vi "AGG MISURE EL NM.vi"(6 "ACQ RESISTOMAT?":bool=TRUE, 7 "Cluster INFO":T26={"Scelta wattmetro"={"Wattmetro"=enum."No Selection"}, "SET RPM"=0.0, "SET TEMP"=0.0, "Array banchi"=[{"Nome"="Elettropompa", "Tors. scala1"=0, "Tors. scala2"=0, "rpm"=0, "TAMB"=0, "Indici Temperature"=[0, 1], "Indice freno"=1, "alimentatore trifase"=0, "alimentatore monofase"=0, "alimentatore dc arm"=0, "alimentatore dc ecc"=0, "alimentatore dc mp"=0}, {"Nome"="Sommersa", "Tors. scala1"=0, "Tors. scala2"=0, "rpm"=0, "TAMB"=1, "Indici Temperature"=[0, 1], "Indice freno"=0, "alimentatore trifase"=0, "alimentatore monofase"=0, "alimentatore dc arm"=0, "alimentatore dc ecc"=0, "alimentatore dc mp"=0}], "Array valvole linee avvio/fermata"=[], "banco selezionato"=0, "Nomi valvole prop sistema"=[], "canale-- sensore"=[], "Attriti B1"=[], "Attriti B2"=[], "Collegamento elettrico"={"ALIMENTAZIONE ELETTRICA"=enum."AC TRIFASE", "ID"=0, "#rami freddo\\eq term resmeter"=0, "#rami riscaldamento resmeter"=0, "#rami freddo\\eq term resistomat"=0, "#rami riscaldamento resistomat"=0, "CALCOLI"=enum."AC TRIFASE"}, "lingua"=0, "Costanti collaudo"={"P [bar]"=0.0, "T amb. [°C]"=0.0, "Umidità [%]"=0.0, "T acqua [°C] 2"=0.0}, "OPZIONI MISURE RES"={"MISURA A FREDDO"=enum."RESISTOMAT", "MISURA EQ. TERMICO"=enum."RESISTOMAT", "MISURA DT PROVA IN CORSO"=enum."RESISTOMAT - CON FERMATE", "MISURE PRIMA E DOPO"=enum."RESISTOMAT", "STRUMENTI PRESENTI"=enum."NESSUNO"}, "Dati targa motore"={"Vnom"=0.0, "Fnom"=0.0, "Inom"=0.0, "Cnom"=0.0, "Npoli"=0.0, "Scorta 1"=0.0, "Scorta 2"=0.0, "Scorta 3"=0.0}}, 8 "RPM":dbl, 9 "tamb":dbl format="%#_13g", 10 "MISURE ALL":T1={"Cluster READ NI"={"AI (0-10V)"={"AI 0"=0.0, "AI 1"=0.0, "AI 2"=0.0, "AI 3"=0.0, "AI 4"=0.0, "AI 5"=0.0, "AI 6"=0.0, "AI 7"=0.0, "AI 8"=0.0, "AI 9"=0.0, "AI 10"=0.0, "AI 11"=0.0, "AI 12"=0.0, "AI 13"=0.0, "AI 14"=0.0, "AI 15"=0.0, "AI 16"=0.0, "AI 17"=0.0, "AI 18"=0.0, "AI 19"=0.0, "AI 20"=0.0, "AI 21"=0.0, "AI 22"=0.0, "AI 23"=0.0, "AI 24"=0.0, "AI 25"=0.0, "AI 26"=0.0, "AI 27"=0.0, "AI 28"=0.0, "AI 29"=0.0, "AI 30"=0.0, "AI 31"=0.0}, "StatoAO_Cdaq[0-10V]"={"AO 1"=0.0, "AO 2"=0.0, "AO 3"=0.0, "AO 4"=0.0}, "Contatori [rpm]"={"RPM 1"=0.0, "RPM 2"=0.0}, "StatoAO_Cdaq [4-20mA]"={"Cdaq_AO [0-10V] 0 for Torque"=0.0, "Cdaq_AO [0-10V] 1"=0.0, "Cdaq_AO [0-10V] 2"=0.0, "Cdaq_AO [0-10V] 3"=0.0}, "StatoDO_Cdaq"={"Scorta 0"=FALSE, "Scorta 1"=FALSE, "Scorta 2"=FALSE, "Scorta 3"=FALSE, "Scorta 4"=FALSE, "Scorta 5"=FALSE, "Scorta 6"=FALSE, "Scorta 7"=FALSE, "Scorta 8"=FALSE, "Scorta 9"=FALSE, "Scorta 10"=FALSE, "Scorta 11"=FALSE, "Scorta 12"=FALSE, "Scorta 13"=FALSE, "Scorta 14"=FALSE, "Scorta 15"=FALSE, "Scorta 16"=FALSE, "Scorta 17"=FALSE, "Scorta 18"=FALSE, "Scorta 19"=FALSE, "Scorta 20"=FALSE, "Scorta 21"=FALSE, "Scorta 22"=FALSE, "Scorta 23"=FALSE, "Scorta 24"=FALSE, "Scorta 25"=FALSE, "Scorta 26"=FALSE, "Scorta 27"=FALSE, "Scorta 28"=FALSE, "Scorta 29"=FALSE, "Scorta 30"=FALSE, "Scorta 31"=FALSE}, "DI"={"Scorta 0"=FALSE, "Scorta 1"=FALSE, "Scorta 2"=FALSE, "Scorta 3"=FALSE, "Scorta 4"=FALSE, "Scorta 5"=FALSE, "Scorta 6"=FALSE, "Scorta 7"=FALSE, "Scorta 8"=FALSE, "Scorta 9"=FALSE, "Scorta 10"=FALSE, "Scorta 11"=FALSE, "Scorta 12"=FALSE, "Scorta 13"=FALSE, "Scorta 14"=FALSE, "Scorta 15"=FALSE, "Scorta 16"=FALSE, "Scorta 17"=FALSE, "Scorta 18"=FALSE, "Scorta 19"=FALSE, "Scorta 20"=FALSE, "Scorta 21"=FALSE, "Scorta 22"=FALSE, "Scorta 23"=FALSE, "Scorta 24"=FALSE, "Scorta 25"=FALSE, "Scorta 26"=FALSE, "Scorta 27"=FALSE, "Scorta 28"=FALSE, "Scorta 29"=FALSE, "Scorta 30"=FALSE, "Scorta 31"=FALSE}, "AI (4-20mA)"={"AI 0"=0.0, "AI 1"=0.0, "AI 2"=0.0, "AI 3"=0.0, "AI 4"=0.0, "AI 5"=0.0, "AI 6"=0.0, "AI 7"=0.0, "AI 8"=0.0, "AI 9"=0.0, "AI 10"=0.0, "AI 11"=0.0, "AI 12"=0.0, "AI 13"=0.0, "AI 14"=0.0, "AI 15"=0.0}, "TC [°C]"={"tc 1"=0.0, "tc 2"=0.0, "tc 3"=0.0, "tc 4"=0.0}, "NI Read Values"={"RPM"=0.0, "Frequency"=0.0, "Mod 1"={"Torsiometro 1"=0.0, "Torsiometro 2"=0.0, "Strin Gauge 1"=0.0, "Strin Gauge 2"=0.0}, "Mod 2"={"Termocoppia 1"=0.0, "Termocoppia 2"=0.0, "Termocoppia 3"=0.0, "Termocoppia 4"=0.0}, "Mod 3"={"PT 100 1"=0.0, "PT 100 2"=0.0, "PT 100 3"=0.0, "PT 100 4"=0.0}}}, "MISURE WT"={"URMS 1"=0.0, "IRMS 1"=0.0, "P 1"=0.0, "S 1"=0.0, "Q 1"=0.0, "LAMBDA 1"=0.0, "PHI 1"=0.0, "F U 1"=0.0, "F I 1"=0.0, "NONE 1"=0.0, "URMS 2"=0.0, "IRMS 2"=0.0, "P 2"=0.0, "S 2"=0.0, "Q 2"=0.0, "LAMBDA 2"=0.0, "PHI 2"=0.0, "F U 2"=0.0, "F I 2"=0.0, "NONE 2"=0.0, "URMS 3"=0.0, "IRMS 3"=0.0, "P 3"=0.0, "S 3"=0.0, "Q 3"=0.0, "LAMBDA 3"=0.0, "PHI 3"=0.0, "F U 3"=0.0, "F I 3"=0.0, "NONE 3"=0.0, "URMS SIGMA"=0.0, "IRMS SIGMA"=0.0, "P SIGMA"=0.0, "S SIGMA"=0.0, "Q SIGMA"=0.0, "LAMBDA SIGMA"=0.0, "PHI SIGMA"=0.0, "F U SIGMA"=0.0, "F I SIGMA"=0.0, "NONE 4"=0.0}, "Resistenze Resistomat"={"Res Ch1"=0.0, "Res Ch2"=0.0, "Res Ch3"=0.0, "Tamb"=0.0}, "INTERFACCIA"={"AI"={"Portate"=[], "Pressioni"=[], "Coppie[Nm]"=[], "Valvole prop %"=[], "RPM"=[], "Livelli"=[], "Temperature"=[], "Riferimenti %"=[], "TENSIONI"=[], "CORRENTI"=[]}, "DI (logici)"={"Start da pulsantiera"=FALSE, "Stop da pulsantiera"=FALSE, "Reset da pulsantiera"=FALSE, "Sistema OK"=FALSE, "Collaudo abilitato"=FALSE, "Potenza trifase abilitata"=FALSE, "Potenza monofase abilitata"=FALSE, "Potenza DC abilitata"=FALSE, "Potenza DC ECC abilitata"=FALSE, "Start alimentazione AC"=FALSE, "Start alimentazione DC"=FALSE, "Start DC eccitazione"=FALSE, "Teleruttore WT abilitato"=FALSE, "Teleruttore Resistomat abilitato"=FALSE, "Teleruttore corto fasi"=FALSE, "Ramo 1 resistomat"=FALSE, "Ramo 2 resistomat"=FALSE, "Ramo 3 resistomat"=FALSE, "B1 Scelta linea elettrica 1"=FALSE, "B1 Scelta linea elettrica 2"=FALSE, "B1 Scelta linea elettrica 3"=FALSE, "B1 Scelta linea elettrica 4"=FALSE, "B1 Scelta linea elettrica 5"=FALSE, "B2 Scelta linea elettrica 1"=FALSE, "B2 Scelta linea elettrica 2"=FALSE, "B2 Scelta linea elettrica 3"=FALSE, "B2 Scelta linea elettrica 4"=FALSE, "B2 Scelta linea elettrica 5"=FALSE, "Rotore bloccato 1"=FALSE, "Rotore bloccato 2"=FALSE, "FRENO 1 abilitato"=FALSE, "FRENO 1 run"=FALSE, "FRENO 1 senso rotaz"=FALSE, "FRENO 1 ctrl velocità"=FALSE, "FRENO 2 abilitato"=FALSE, "FRENO 2 run"=FALSE, "FRENO 2 senso rotaz"=FALSE, "FRENO 2 ctrl velocità"=FALSE, "ALIM 1 abilitato"=FALSE, "ALIM 1 run"=FALSE, "ALIM 2 abilitato"=FALSE, "ALIM 2 run"=FALSE, "ALIM 3 abilitato"=FALSE, "ALIM 3 run"=FALSE, "FRENO 1 ctrl coppia"=FALSE, "FRENO 2 ctrl coppia"=FALSE, "FRENO 3 ctrl coppia"=FALSE, "DI (logici) aggiuntivi impianto"={"Solo freno abilitato"=FALSE, "Carico resistivo abilitato"=FALSE, "AFE+freno abilitato"=FALSE, "Protezioni chiuse"=FALSE, "Start potenza AFE"=FALSE, "AFE in marcia"=FALSE}, "Misura corrente diretta WT"=FALSE, "Misura corrente sens ext"=FALSE, "Sens ext abilitati"=FALSE}, "AO non scalati"={"FRENO1 rif vel"=0.0, "FRENO1 rif Coppia"=0.0, "FRENO2 rif vel"=0.0, "FRENO2 rif Coppia"=0.0, "ALIM1 rif V"=0.0, "ALIM1 rif F"=0.0, "ALIM2 rif V"=0.0, "ALIM2 rif F"=0.0, "ALIM3 rif V"=0.0, "ALIM3 rif F"=0.0, "Fnom keb"=0.0, "Rpm nom keb"=0.0, "Pnom keb"=0.0, "Inom keb"=0.0, "Vnom keb"=0.0, "Rpm max keb"=0.0, "Tempo rampa keb"=0.0, "Tipo Mot keb"=0.0, "FRENO  rif Coppia "=0.0, "FRENO  rif  Corrente"=0.0}, "AO scalati"={"FRENO1 rif vel"=0.0, "FRENO1 rif Coppia"=0.0, "FRENO2 rif vel"=0.0, "FRENO2 rif Coppia"=0.0, "ALIM1 rif V"=0.0, "ALIM1 rif F"=0.0, "ALIM2 rif V"=0.0, "ALIM2 rif F"=0.0, "ALIM3 rif V"=0.0, "ALIM3 rif F"=0.0, "Fnom keb"=0.0, "Rpm nom keb"=0.0, "Pnom keb"=0.0, "Inom keb"=0.0, "Vnom keb"=0.0, "Rpm max keb"=0.0, "Tempo rampa keb"=0.0, "Tipo Mot keb"=0.0, "FRENO  rif Coppia "=0.0, "FRENO  rif  Corrente"=0.0}, "DO (logici)"={"Scelta banco 1"=FALSE, "Scelta banco 2"=FALSE, "Scelta banco 3"=FALSE, "FRENO 1 abilita"=FALSE, "FRENO 1 start"=FALSE, "FRENO 1 senso rotaz"=FALSE, "FRENO 1 ctrl velocità"=FALSE, "FRENO 2 abilita"=FALSE, "FRENO 2 start"=FALSE, "FRENO 2 senso rotaz"=FALSE, "FRENO 2 ctrl velocità"=FALSE, "ALIM 1 abilita"=FALSE, "ALIM 1 start"=FALSE, "ALIM 2 abilita"=FALSE, "ALIM 2 start"=FALSE, "ALIM 3 abilita"=FALSE, "ALIM 3 start"=FALSE, "Abilita linea trifase"=FALSE, "Abilita linea monofase"=FALSE, "Abilita linea dc"=FALSE, "Abilita linea dc eccit"=FALSE, "B1 Linea elettrica 1"=FALSE, "B1 Linea elettrica 2"=FALSE, "B1 Linea elettrica 3"=FALSE, "B1 Linea elettrica 4"=FALSE, "B1 Linea elettrica 5"=FALSE, "B2 Linea elettrica 1"=FALSE, "B2 Linea elettrica 2"=FALSE, "B2 Linea elettrica 3"=FALSE, "B2 Linea elettrica 4"=FALSE, "B2 Linea elettrica 5"=FALSE, "Start potenza AC"=FALSE, "Stop pontenza AC"=FALSE, "Start potenza DC"=FALSE, "Stop potenza DC"=FALSE, "Start potenza eccitaz"=FALSE, "Stop potenza eccitaz"=FALSE, "Reset allarmi"=FALSE, "watchdog"=FALSE, "Scala torsiometro B1"=FALSE, "Controllo torsiom B1"=FALSE, "Scala torsiometro B2"=FALSE, "Controllo torsiom B2"=FALSE, "Teleruttore WT abilita"=FALSE, "Teleruttore Resistomat abilita"=FALSE, "Teleruttore corto fasi"=FALSE, "Ramo 1 resistomat"=FALSE, "Ramo 2 resistomat"=FALSE, "Ramo 3 resistomat"=FALSE, "Collaudo in corso"=FALSE, "Allarme presente"=FALSE, "Enable Res Meter"=FALSE, "Bypass Res Meter"=FALSE, "2nd canale Res Meter"=FALSE, "Scala 200/2000 res meter"=FALSE, "Taratura res meter"=FALSE, "FRENO 1 ctrl coppia"=FALSE, "FRENO 2 ctrl coppia"=FALSE, "FRENO 3 ctrl coppia"=FALSE, "Aggiuntivi impianto"={"Senso rotazione alim 1"=FALSE, "Senso rotazione alim 2"=FALSE}, "ALIM 1 stop"=FALSE, "ALIM 2 stop"=FALSE, "ALIM 3 stop"=FALSE, "FRENO 1 stop"=FALSE, "FRENO 2 stop"=FALSE, "FRENO 3 stop"=FALSE, "B1 configurazione freno B"=FALSE, "B2 configurazione freno B"=FALSE, "Abilita scrittura KEB"=FALSE, "Bench Selection (0-B1,1-B2)"=FALSE, "Select current mode"=FALSE, "Select torque mode"=FALSE, "Select speed mode"=FALSE, "Start"=FALSE, "Stop"=FALSE, "Block"=FALSE, "Enable Force mode"=FALSE, "Abilita linea 125 A"=FALSE, "Abilita linea 63 A"=FALSE, "Abilita linea 16 A"=FALSE, "Aum Tensione Variac"=FALSE, "Dim Tesnione Variac"=FALSE, "Abilita ellectro stractura"=FALSE, "Risprinito Emergence"=FALSE, "Abilita collaudo"=FALSE, "Disabilita collaudo"=FALSE, "External Alaram"=FALSE, "Enable external program"=FALSE, "Reset"=FALSE, "Abilita Ingresso Variac"=FALSE, "Abilita Ventilatore Variac"=FALSE, "Abilita Uscita Variac "=FALSE}}, "FREDDO resistomat"={"Res Ch1"=0.0, "Res Ch2"=0.0, "tAMB"=0.0, "Res Ch3"=0.0}, "STATO PLC 1"={"USCITE PLC"={"AO (real) 2"={"SCORTA 1"=0.0, "SCORTA 2"=0.0, "SCORTA 3"=0.0, "SCORTA 4"=0.0, "SCORTA 5"=0.0, "SCORTA 6"=0.0, "SCORTA 7"=0.0, "SCORTA 8"=0.0}, "statoAO_PLC out"={"Rif Lim coppia freno [%]"=nan, "Rif rpm freno [%]"=nan, "Rif coppia freno [%]"=0.0, "Rif V alimentatore [%]"=0.0, "Rif F alimentatore [%]"=0.0}, "DO (bit)"={"Scelta banco 1"=FALSE, "Set dati motore freno 2"=FALSE, "Diretto inverter"=FALSE, "Filtro LC"=FALSE, "Marcia ALIM (1s)"=FALSE, "Marcia FRENO (1s)"=FALSE, "Stop AFE (1s)"=FALSE, "Stop freno (1s)"=FALSE, "Reset allarmi"=FALSE, "Watchdog"=FALSE, "Senso rotazione"=FALSE, "Abilita collaudo (1s)"=FALSE, "Disabilita collaudo (1s)"=FALSE, "Abilitazione ALIM"=FALSE, "Abilitazione FRENO"=FALSE, "Teleruttore WT"=FALSE, "Senso rot motore prova"=FALSE, "Scorta 7"=FALSE, "Scorta 8"=FALSE, "Scorta 9"=FALSE, "Scorta 10"=FALSE, "Scorta 11"=FALSE, "Scorta 12"=FALSE, "Scorta 13"=FALSE}}, "Stato DI_PLC"={"Sistema OK"=FALSE, "Rotore bloccato"=FALSE, "Scorta 1"=FALSE, "Prova diretto inverter"=FALSE, "Prova con filtro LC"=FALSE, "Teleruttore WT abilitato"=FALSE, "Alim sinus penta abilitato"=FALSE, "Alim sinus penta in marcia"=FALSE, "Freno abilitato"=FALSE, "Freno in marcia"=FALSE, "Senso rotazione freno"=FALSE, "Potenza abilitata"=FALSE, "Scorta 3"=FALSE, "Scorta 4"=FALSE, "scorta 5"=FALSE, "scorta 6"=FALSE}, "AI plc"={"Allarmi 1"=0.0, "Allarmi 2"=0.0, "Scorta 1"=0.0, "Scorta 2"=0.0, "RPM mot prova"=0.0, "I mot prova"=0.0, "RPM freno"=0.0, "I freno"=0.0, "Scorta 3"=0.0, "Scorta 4"=0.0}}, "Res Ch2"=0.0, "Res Ch2 2"=0.0, "FREDDO res meter"={"Res Ch1"=0.0, "Res Ch2"=0.0, "tAMB"=0.0, "Res Ch3"=0.0}, "Resistenze Res Meter"={"Res Ch1"=0.0, "Res Ch2"=0.0, "Res Ch3"=0.0, "Tamb"=0.0}, "READ SINUS PENTA"={"Menù Misure motore (M000-M030)"={"Rif vel a regime (int)"=0, "Rif vel a regime (dec)"=0, "Rif vel dopo rampe (int)"=0, "Rif vel dopo rampe (dec)"=0, "RPM motore (int)"=0, "RPM motore (dec)"=0, "FREQout inverter"=0, "Rif coppia a regime(Nm)"=0, "Richiesta di coppia (Nm)"=0, "Coppia generata dal motore(Nm)"=0, "Rif coppia a regime(%)"=0, "Richiesta di coppia (%)"=0, "Coppia generata dal motore(%)"=0, "Coppia max richiesta prima delle rampe(Nm)"=0, "Coppia max richiesta dopo le rampe(Nm)"=0, "Limite di velocità prima delle rampe"=0, "Limite di velocità dopo le rampe"=0, "Coppia max richiesta prima delle rampe(%)"=0, "Coppia max richiesta dopo le rampe(%)"=0, "Rif di flusso"=0, "Corrente di uscita"=0, "Capacità termica del motore"=0, "Tensione di uscita"=0, "Potenza di uscita"=0, "Energia consumata (LSword)"=0, "Energia consumata (MSword)"=0, "Tensione bus DC"=0, "Tensione di rete"=0}, "Menù regolatore PID (M018-M024)"={"Rif PID a regime(%)"=0, "Rif pid dopo rampe(%)"=0, "Retroazione del pid(%)"=0, "Errore del pid(%)"=0, "uscita del pid(%)"=0, "Rif del pid dopo le rampe"=0, "Retroazione del pid"=0}, "Menù ingressi digitali (M031-M036)"={"Ingressi digitali ritardati"=0, "Ingressi digitali istantanei"=0, "Moresettiera comando loc"=0, "Morsett comando da seriale"=0, "Morsett comando bus di campo"=0, "Ing dig ausiliari da morsettiera"=0, "Ing dig ausiliari da seriale"=0}, "Menù riferimenti (M037-M051)"={"Rif analog est REF"=0, "Rif analog est AIN1"=0, "Rif analog est AIN2"=0, "Rif analog est XAIN4"=0, "Rif analog est XAIN5"=0, "Rif velocità da seriale(int)"=0, "Rif velocità bus di campo(int)"=0, "Rif coppia da seriale"=0, "Rif coppia bus di campo"=0, "Rif del PID da seriale"=0, "Rif del PID da bus di campo"=0, "Retroazione del PID da seriale"=0, "Retroazione del PIDda bus di campo"=0, "Rif da encoder"=0, "Rif in frequenza"=0, "Rif velocità da seriale(dec)"=0, "Rif velocità bus di campo(dec)"=0}, "Menù rampe (P009-P033)"={"Tempo di dec rampa di vel 1"=0, "Tempo di acc rampa di vel 2"=0, "Tempo di dec rampa di vel 2"=0, "Tempo di acc rampa di vel 1"=0, "Unità di mis tempi rampe vel 1/2"=0, "Tempo di acc rampa di vel 3"=0, "Tempo di dec rampa di vel 3"=0, "Tempo di acc rampa di vel 4"=0, "Tempo di dec rampa di vel 4"=0, "Unità di mis tempi rampe vel 3/4"=0, "Selettore arrottondam rampe"=0, "Tempo di arrotond iniz rampa acc"=0, "Tempo di arrotond finale rampa acc"=0, "Tempo di arrotond iniz rampa dec"=0, "Tempo di rampa di salita rif coppia"=0, "Tempo di rampa di discesa rif coppia"=0, "Unità di misura rampa coppia"=0, "Tempo rampa acc marcia jog"=0, "Tempo rampa dec marcia jog"=0, "Reset acc ai cambi pendenza"=0, "rampa di acc in fire mode"=0, "rampa di dec in fire mode"=0, "Tempo di arrotond finale rampa dec"=0}, "Menù controllo motore(C008-C128)"={"Numero motori configurati"=0, "Tipo algoritmo di controllo Mot1"=0, "Tipo rif Mot1"=0, "Tensione nominale rete"=0, "Retroaz di vel da encoder Mot1"=0, "Tipo curva V/f Mot1"=0, "Rotazione delle fasi Mot1"=0, "Freq nominale del motore Mot1"=0, "RPM nominali del motore Mot1"=0, "Potenza nominale del motore Mot1"=0, "Corrente nominale del motore Mot1"=0, "Tensione nominale del motore mot1"=0, "Potenza a vuoto del motore Mot1"=0, "Corrente a vuoto del motore Mot1"=0, "Resistenza statorica del motore Mot1"=0, "Induttanza di dispersione Mot1"=0, "Induttanza mutua motore"=0, "Costante di tempo rotorica"=0, "Costante di tempo filtro pb"=0, "Velocità minima motore"=0, "Velocità massima motore"=0}, "Menù configurazione PID"={"Selezione riferimento n.1"=0, "Selezione retroazione n.1"=0, "Modalità di fuzionamento PID"=0, "Termine derivativo calcolato su err o mis"=0, "Proporz moltiplica deriv e integrale"=0, "Azione del PID"=0}, "ID"=0.0, "Menù uscite digitali"={"MDO4 Inverter pronto"=0}, "Fcarrier"={"Fcarrier Min (Hz)"=0, "Fcarrier Max (Hz)"=0}, "stato inverter M089"=0.0, "Riferimenti"={"Rif tensione"=0, "Rif velocità"=0}, "Comunicazione"=FALSE, "Modalità stop"=0.0}, "STATO PLC 2"={"USCITE PLC"={"AO (real) 2"={"SCORTA 1"=0.0, "SCORTA 2"=0.0, "SCORTA 3"=0.0, "SCORTA 4"=0.0, "SCORTA 5"=0.0, "SCORTA 6"=0.0, "SCORTA 7"=0.0, "SCORTA 8"=0.0}, "statoAO_PLC out"={"Condensatori"=0.0, "Scorta 1"=0.0, "Scorta 2"=0.0}, "DO (bit)"={"Relè misura resistomat"=FALSE, "Misura res ramo 1"=FALSE, "Misura res ramo 2"=FALSE, "Misura res ramo 3"=FALSE, "Scelta banco 2"=FALSE, "Scala Torsiometro"=FALSE, "Ctrl torsiometro"=FALSE, "Select current mode"=FALSE, "Select Torque mode"=FALSE, "Select speed mode"=FALSE, "Watchdog"=FALSE, "Scorta"=FALSE, "Scorta 2"=FALSE, "Scorta 3"=FALSE, "Scorta 4"=FALSE, "Scorta 5"=FALSE, "Bench selection"=FALSE, "External alarm"=FALSE, "Enable external program"=FALSE, "Reset allarmi"=FALSE, "Start"=FALSE, "Stop"=FALSE, "Block"=FALSE, "Scorta 6"=FALSE}}, "Stato DI_PLC"={"Sistema ok"=FALSE, "Relè Resistomat abilitato"=FALSE, "Freno abilitato"=FALSE, "Freno in marcia"=FALSE, "scorta b"=FALSE, "scorta a"=FALSE, "scorta 1"=FALSE, "scorta 2"=FALSE, "scorta 3"=FALSE, "scorta 4"=FALSE, "Scorta 5"=FALSE, "Scorta 6"=FALSE, "Scorta 7"=FALSE, "Scorta 8"=FALSE, "Scorta 9"=FALSE, "Scorta 10"=FALSE}, "AI plc"={"Allarmi 1"=0.0, "Allarmi 2"=0.0, "TC 1"=0.0, "TC 2"=0.0, "TC 3"=0.0, "TC 4"=0.0, "TC 5"=0.0, "TC 6"=0.0, "TC 7"=0.0, "TC 8"=0.0, "PT1000 1"=0.0, "PT1000 2"=0.0, "PT1000 3"=0.0, "PT1000 4"=0.0}}, "STATO PLC 3"={"USCITE PLC"={"AO (real) 2"={"SCORTA 1"=0.0, "SCORTA 2"=0.0, "SCORTA 3"=0.0, "SCORTA 4"=0.0, "SCORTA 5"=0.0, "SCORTA 6"=0.0, "SCORTA 7"=0.0, "SCORTA 8"=0.0}, "statoAO_PLC out"={"Rif velocità alimentatore"=0.0, "Scorta"=0.0, "Tipo Motore  keb"=0.0, "I nom keb"=0.0, "RPM nom keb"=0.0, "V nom keb"=0.0, "F nom keb"=0.0, "t rampa keb"=0.0}, "DO (bit)"={"Select linea Inverter"=FALSE, "Abilita sense wattmetro"=FALSE, "Bypass filtro LC"=FALSE, "Filtro LC"=FALSE, "Bypass trasformatore"=FALSE, "Trasformatore"=FALSE, "Abilita uscite variac"=FALSE, "Abilita linea 125 A"=FALSE, "Abilita linea 63 A"=FALSE, "Abilita linea 16 A"=FALSE, "Abilita Scrittura Dati Keb"=FALSE, "Abilita alimentatore"=FALSE, "Marcia alimentatore (1s)"=FALSE, "Stop alimentatore (1s)"=FALSE, "Senso rot mot prova"=FALSE, "Watchdog"=FALSE, "Aumenta tensione variac"=FALSE, "Diminuisci tensione variac "=FALSE, "Blocco elettroserrature"=FALSE, "Ripristino emergence"=FALSE, "Abilita ingresso variac"=FALSE, "Abilita ventilatore variac"=FALSE, "Reset Allarm"=FALSE, "Scorta 1"=FALSE, "Scorta 2"=FALSE, "Scorta 3"=FALSE, "Scorta 4"=FALSE, "Scorta 5"=FALSE, "Scorta 6"=FALSE, "Scorta 7"=FALSE, "Scorta 8"=FALSE, "Scorta 9"=FALSE, "Abilita collaudo"=FALSE, "Disabilita collaudo "=FALSE, "Scorta 10"=FALSE, "Scorta 11"=FALSE, "Scorta 12"=FALSE, "Scorta 13"=FALSE, "Scorta 14"=FALSE, "Scorta 15"=FALSE}}, "Stato DI_PLC"={"Sistema OK"=FALSE, "Rotore bloccato"=FALSE, "Filtro LC"=FALSE, "Bypass Filtro LC"=FALSE, "Scelta Trasformatore"=FALSE, "Scelta Bypass trasformatore"=FALSE, "Teleruttore wt abilitato"=FALSE, "Alimentatore abilitato"=FALSE, "Alimentatore in marcia"=FALSE, "Scorta 1"=FALSE, "Scorta 2"=FALSE, "Scorta 3"=FALSE, "Potenza abilitata"=FALSE, "Alimentatore in allarme"=FALSE, "Scorta 4"=FALSE, "Conferma dati KEB"=FALSE, "Scorta 5"=FALSE, "Warning Inverter Alimentatore"=FALSE, "Variac Abilitato"=FALSE, "Linea 125 A abilitata"=FALSE, "Linea 63 A abilitata"=FALSE, "Linea 16 A abilitata"=FALSE, "Scorta 6"=FALSE, "Enable force mode"=FALSE}, "AI plc"={"Allarmi 1"=0.0, "Allarmi 2"=0.0, "RPM motore prova"=0.0, "Corrente motore prova"=0.0, "RPM freno"=0.0, "Corrente freno"=0.0, "Tipo motore keb"=0.0, "I nom keb"=0.0, "RPM nom keb"=0.0, "V nom keb"=0.0, "F nom keb"=0.0, "T rampa keb"=0.0, "scorta"=0.0, "Scorta 2"=0.0}}, "DCREG"={"Parametri di misura"={"M000"=0.0, "M001"=0.0, "M002"=0.0, "M003"=0.0, "M004"=0.0, "M005"=0.0, "M006"=0.0, "M007"=0.0, "M008"=0.0, "M009"=0.0, "M010"=0.0, "M011"=0.0, "M012"=0.0, "M013"=0.0, "M014"=0.0, "M015"=0.0, "M016"=0.0, "M017"=0.0, "M018"=0.0, "M019"=0.0, "M020"=0.0, "M021"=0.0, "M022"=0.0, "M023"=0.0, "M024"=0.0, "M025"=0.0, "M026"=0.0, "M027"=0.0, "M028"=0.0, "M029"=0.0, "M030"=0.0, "M031"=0.0}, "Parametri di programmazione"={"P000"=0.0, "P001"=0.0, "P002"=0.0, "P003"=0.0, "P004"=0.0, "P005"=0.0, "P006"=0.0, "P010"=0.0, "P011"=0.0, "P012"=0.0, "P013"=0.0, "P014"=0.0, "P015"=0.0, "P016"=0.0, "P030"=0.0, "P031"=0.0, "P032"=0.0, "P033"=0.0, "P034"=0.0, "P035"=0.0, "P036"=0.0, "P037"=0.0, "P038"=0.0, "P039"=0.0, "P040"=0.0, "P050"=0.0, "P051"=0.0, "P052"=0.0, "P053"=0.0, "P054"=0.0, "P055"=0.0, "P056"=0.0, "P057"=0.0, "P058"=0.0, "P059"=0.0, "P060"=0.0, "P061"=0.0, "P062"=0.0, "P070"=0.0, "P071"=0.0, "P073"=0.0, "P074"=0.0, "P076"=0.0, "P077"=0.0, "P079"=0.0, "P080"=0.0, "P082"=0.0, "P083"=0.0, "P084"=0.0, "P085"=0.0, "P086"=0.0, "P087"=0.0, "P088"=0.0, "P100"=0.0, "P101"=0.0, "P102"=0.0, "P103"=0.0, "P104"=0.0, "P110"=0.0, "P111"=0.0, "P120"=0.0, "P121"=0.0, "P122"=0.0, "P123"=0.0, "P124"=0.0, "P125"=0.0, "P126"=0.0, "P127"=0.0, "P128"=0.0, "P129"=0.0, "P130"=0.0, "P131"=0.0, "P132"=0.0, "P133"=0.0, "P134"=0.0, "P150"=0.0, "P151"=0.0, "P152"=0.0, "P153"=0.0, "P154"=0.0, "P155"=0.0, "P156"=0.0, "P157"=0.0, "P158"=0.0, "P170"=0.0, "P171"=0.0, "P172"=0.0, "P173"=0.0, "P174"=0.0, "P175"=0.0, "P176"=0.0, "P177"=0.0, "P178"=0.0, "P179"=0.0, "P180"=0.0, "P181"=0.0, "P182"=0.0, "P183"=0.0, "P184"=0.0, "P185"=0.0, "P186"=0.0, "P187"=0.0, "P188"=0.0, "P189"=0.0, "P190"=0.0, "P191"=0.0, "P192"=0.0, "P193"=0.0, "P194"=0.0, "P195"=0.0, "P196"=0.0, "P197"=0.0, "P198"=0.0, "P199"=0.0, "P211"=0.0, "P212"=0.0, "P213"=0.0, "P214"=0.0, "P215"=0.0, "P216"=0.0, "P217"=0.0, "P221"=0.0, "P222"=0.0, "P223"=0.0, "P224"=0.0, "P230"=0.0, "P231"=0.0, "P240"=0.0, "P250"=0.0, "P251"=0.0}, "Parametri di configurazione"={"C000"=0.0, "C001"=0.0, "C002"=0.0, "C010"=0.0, "C011"=0.0, "C012"=0.0, "C014"=0.0, "C015"=0.0, "C016"=0.0, "C017"=0.0, "C018"=0.0, "C030"=0.0, "C050"=0.0, "C051"=0.0, "C052"=0.0, "C060"=0.0, "C061"=0.0, "C062"=0.0, "C063"=0.0, "C070"=0.0, "C072"=0.0, "C074"=0.0, "C090"=0.0, "C091"=0.0, "C092"=0.0, "C093"=0.0, "C094"=0.0, "C100"=0.0, "C101"=0.0, "C102"=0.0, "C103"=0.0, "C105"=0.0, "C106"=0.0, "C107"=0.0, "C108"=0.0, "C110"=0.0, "C111"=0.0, "C112"=0.0, "C120"=0.0, "C121"=0.0, "C122"=0.0, "C130"=0.0, "C131"=0.0, "C132"=0.0, "C133"=0.0, "C134"=0.0, "C135"=0.0, "C141"=0.0, "C142"=0.0, "C143"=0.0, "C150"=0.0, "C151"=0.0, "C153"=0.0, "C154"=0.0, "C155"=0.0, "C156"=0.0, "C157"=0.0, "C158"=0.0, "C159"=0.0, "C160"=0.0, "C161"=0.0, "C162"=0.0, "C163"=0.0, "C164"=0.0, "C165"=0.0, "C170"=0.0}, "Codice allarme"=0.0, "Comunicazione"=FALSE}} {"Cluster READ NI"."AI (4-20mA)"."AI 15" format="%#_6f"; "Cluster READ NI"."AI (4-20mA)"."AI 14" format="%#_6f"; "Cluster READ NI"."AI (4-20mA)"."AI 13" format="%#_6f"; "Cluster READ NI"."AI (4-20mA)"."AI 11" format="%#_6f"; "Cluster READ NI"."AI (4-20mA)"."AI 10" format="%#_6f"; "Cluster READ NI"."AI (4-20mA)"."AI 9" format="%#_6f"; "Cluster READ NI"."AI (4-20mA)"."AI 4" format="%#_6f"; "Cluster READ NI"."AI (4-20mA)"."AI 12" format="%#_6f"; "Cluster READ NI"."AI (4-20mA)"."AI 0" format="%#_6f"; "Cluster READ NI"."AI (4-20mA)"."AI 1" format="%#_6f"; "Cluster READ NI"."AI (4-20mA)"."AI 2" format="%#_6f"; "Cluster READ NI"."AI (4-20mA)"."AI 3" format="%#_6f"; "Cluster READ NI"."AI (4-20mA)"."AI 5" format="%#_6f"; "Cluster READ NI"."AI (4-20mA)"."AI 6" format="%#_6f"; "Cluster READ NI"."AI (4-20mA)"."AI 7" format="%#_6f"; "Cluster READ NI"."AI (4-20mA)"."AI 8" format="%#_6f"; "Cluster READ NI"."AI (0-10V)"."AI 31" format="%#_6f"; "Cluster READ NI"."AI (0-10V)"."AI 30" format="%#_6f"; "Cluster READ NI"."AI (0-10V)"."AI 29" format="%#_6f"; "Cluster READ NI"."AI (0-10V)"."AI 28" format="%#_6f"; "Cluster READ NI"."AI (0-10V)"."AI 27" format="%#_6f"; "Cluster READ NI"."AI (0-10V)"."AI 26" format="%#_6f"; "Cluster READ NI"."AI (0-10V)"."AI 25" format="%#_6f"; "Cluster READ NI"."AI (0-10V)"."AI 24" format="%#_6f"; "Cluster READ NI"."AI (0-10V)"."AI 23" format="%#_6f"; "Cluster READ NI"."AI (0-10V)"."AI 22" format="%#_6f"; "Cluster READ NI"."AI (0-10V)"."AI 21" format="%#_6f"; "Cluster READ NI"."AI (0-10V)"."AI 20" format="%#_6f"; "Cluster READ NI"."AI (0-10V)"."AI 19" format="%#_6f"; "Cluster READ NI"."AI (0-10V)"."AI 18" format="%#_6f"; "Cluster READ NI"."AI (0-10V)"."AI 17" format="%#_6f"; "Cluster READ NI"."AI (0-10V)"."AI 16" format="%#_6f"; "Cluster READ NI"."AI (0-10V)"."AI 15" format="%#_6f"; "Cluster READ NI"."AI (0-10V)"."AI 14" format="%#_6f"; "Cluster READ NI"."AI (0-10V)"."AI 13" format="%#_6f"; "Cluster READ NI"."AI (0-10V)"."AI 11" format="%#_6f"; "Cluster READ NI"."AI (0-10V)"."AI 10" format="%#_6f"; "Cluster READ NI"."AI (0-10V)"."AI 9" format="%#_6f"; "Cluster READ NI"."AI (0-10V)"."AI 4" format="%#_6f"; "Cluster READ NI"."AI (0-10V)"."AI 12" format="%#_6f"; "Cluster READ NI"."AI (0-10V)"."AI 0" format="%#_6f"; "Cluster READ NI"."AI (0-10V)"."AI 1" format="%#_6f"; "Cluster READ NI"."AI (0-10V)"."AI 2" format="%#_6f"; "Cluster READ NI"."AI (0-10V)"."AI 3" format="%#_6f"; "Cluster READ NI"."AI (0-10V)"."AI 5" format="%#_6f"; "Cluster READ NI"."AI (0-10V)"."AI 6" format="%#_6f"; "Cluster READ NI"."AI (0-10V)"."AI 7" format="%#_6f"; "Cluster READ NI"."AI (0-10V)"."AI 8" format="%#_6f"}, 11 "MISURE NM in":T31) -> (0 "V":dbl, 3 "MISURE NM out":T31, 4 "P1[W]":dbl)   [LabVIEW 2019]
uses:
  TypeDef/MISURE NM.ctl
  TypeDef/Cluster INFO.ctl
  TypeDef/WT SELECTION.ctl
  TypeDef/Definizione linea.ctl
  TypeDef/Collegamenti_elettrici.ctl
  TypeDef/Control Calcoli.ctl
  TypeDef/Cluster misure ALL.ctl
  TypeDef/Cluster NI.ctl
  cDAQ_PLC Folder/controls/StatoAO_cdaq.ctl
  cDAQ_PLC Folder/controls/statoDO_Cdaq.ctl
  TypeDef/MISURE WT.ctl
  TypeDef/ClusterRes.ctl
  TypeDef/INTERFACCIA.ctl
  TypeDef/Lista AO sistema.ctl
  TypeDef/DOinterfaccia.ctl
  cDAQ_PLC Folder/ST1200_LIST_IO/STATO PLC 1.ctl
  cDAQ_PLC Folder/ST1200_LIST_IO/Uscite PLC 1.ctl
  cDAQ_PLC Folder/controls/statoAO_plc_1.ctl
  cDAQ_PLC Folder/ST1200_LIST_IO/StatoDO_PLC_1.ctl
  SINUS PENTA SANTERNO/controls/Parametri inverter letti.ctl
  cDAQ_PLC Folder/ST1200_LIST_IO/STATO PLC 2.ctl
  cDAQ_PLC Folder/ST1200_LIST_IO/Uscite PLC 2.ctl
  cDAQ_PLC Folder/controls/statoAO_plc_2.ctl
  cDAQ_PLC Folder/ST1200_LIST_IO/StatoDO_PLC_2.ctl
  cDAQ_PLC Folder/ST1200_LIST_IO/STATO PLC 3.ctl
  cDAQ_PLC Folder/ST1200_LIST_IO/Uscite PLC 3.ctl
  cDAQ_PLC Folder/controls/statoAO_plc_3.ctl
  cDAQ_PLC Folder/ST1200_LIST_IO/StatoDO_PLC_3.ctl
  DCREG/Parametri DCREG letti.ctl
  Global DT per visualizzazione.vi
  Global DATI MANUALI.vi
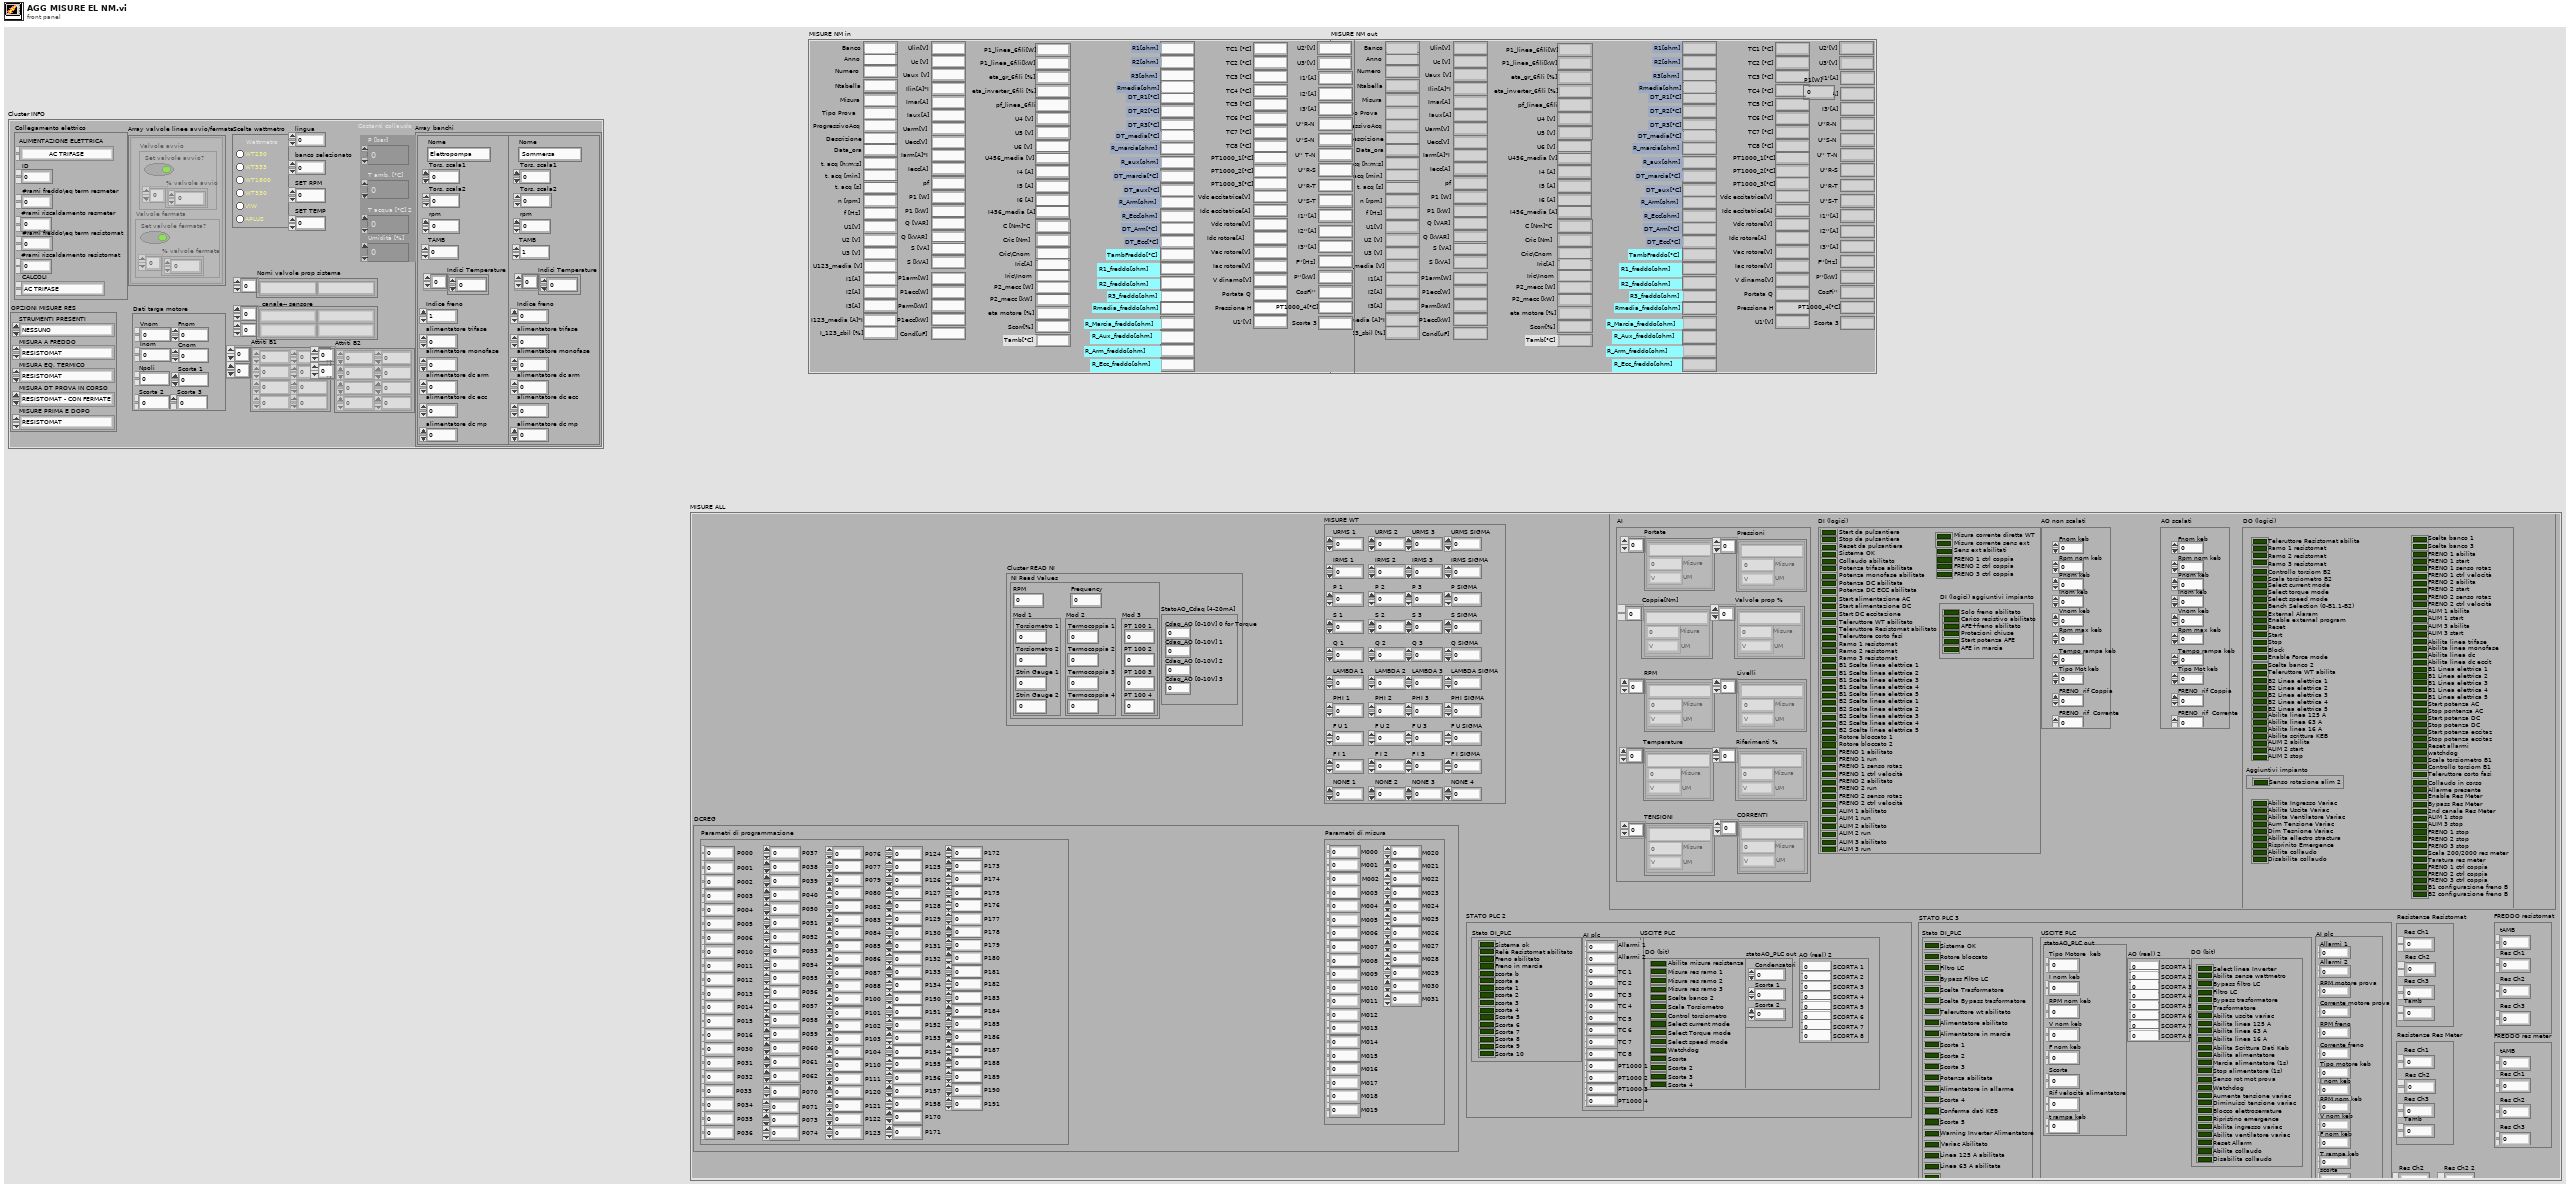
[diagram p1: front panel]
types:
  T1 = typedef "Cluster misure ALL.ctl" = cluster{"Cluster READ NI":T2, "MISURE WT":T5, "Resistenze Resistomat":T6, "INTERFACCIA":T7, "FREDDO resistomat":cluster{"Res Ch1":dbl, "Res Ch2":dbl, "tAMB":dbl, "Res Ch3":dbl}, "STATO PLC 1":T12, "Res Ch2":dbl, "Res Ch2 2":dbl, "FREDDO res meter":cluster{"Res Ch1":dbl, "Res Ch2":dbl, "tAMB":dbl, "Res Ch3":dbl}, "Resistenze Res Meter":T6, "READ SINUS PENTA":T16, "STATO PLC 2":T17, "STATO PLC 3":T21, "DCREG":T25}
  T2 = typedef "Cluster NI.ctl" = cluster{"AI (0-10V)":cluster{"AI 0":dbl, "AI 1":dbl, "AI 2":dbl, "AI 3":dbl, "AI 4":dbl, "AI 5":dbl, "AI 6":dbl, "AI 7":dbl, "AI 8":dbl, "AI 9":dbl, "AI 10":dbl, "AI 11":dbl, "AI 12":dbl, "AI 13":dbl, "AI 14":dbl, "AI 15":dbl, "AI 16":dbl, "AI 17":dbl, "AI 18":dbl, "AI 19":dbl, "AI 20":dbl, "AI 21":dbl, "AI 22":dbl, "AI 23":dbl, "AI 24":dbl, "AI 25":dbl, "AI 26":dbl, "AI 27":dbl, "AI 28":dbl, "AI 29":dbl, "AI 30":dbl, "AI 31":dbl}, "StatoAO_Cdaq[0-10V]":cluster{"AO 1":dbl, "AO 2":dbl, "AO 3":dbl, "AO 4":dbl}, "Contatori [rpm]":cluster{"RPM 1":dbl, "RPM 2":dbl}, "StatoAO_Cdaq [4-20mA]":T3, "StatoDO_Cdaq":T4, "DI":cluster{"Scorta 0":bool, "Scorta 1":bool, "Scorta 2":bool, "Scorta 3":bool, "Scorta 4":bool, "Scorta 5":bool, "Scorta 6":bool, "Scorta 7":bool, "Scorta 8":bool, "Scorta 9":bool, "Scorta 10":bool, "Scorta 11":bool, "Scorta 12":bool, "Scorta 13":bool, "Scorta 14":bool, "Scorta 15":bool, "Scorta 16":bool, "Scorta 17":bool, "Scorta 18":bool, "Scorta 19":bool, "Scorta 20":bool, "Scorta 21":bool, "Scorta 22":bool, "Scorta 23":bool, "Scorta 24":bool, "Scorta 25":bool, "Scorta 26":bool, "Scorta 27":bool, "Scorta 28":bool, "Scorta 29":bool, "Scorta 30":bool, "Scorta 31":bool}, "AI (4-20mA)":cluster{"AI 0":dbl, "AI 1":dbl, "AI 2":dbl, "AI 3":dbl, "AI 4":dbl, "AI 5":dbl, "AI 6":dbl, "AI 7":dbl, "AI 8":dbl, "AI 9":dbl, "AI 10":dbl, "AI 11":dbl, "AI 12":dbl, "AI 13":dbl, "AI 14":dbl, "AI 15":dbl}, "TC [°C]":cluster{"tc 1":dbl, "tc 2":dbl, "tc 3":dbl, "tc 4":dbl}, "NI Read Values":cluster{"RPM":dbl, "Frequency":dbl, "Mod 1":cluster{"Torsiometro 1":dbl, "Torsiometro 2":dbl, "Strin Gauge 1":dbl, "Strin Gauge 2":dbl}, "Mod 2":cluster{"Termocoppia 1":dbl, "Termocoppia 2":dbl, "Termocoppia 3":dbl, "Termocoppia 4":dbl}, "Mod 3":cluster{"PT 100 1":dbl, "PT 100 2":dbl, "PT 100 3":dbl, "PT 100 4":dbl}}}
  T3 = typedef "StatoAO_cdaq.ctl" = cluster{"Cdaq_AO [0-10V] 0 for Torque":dbl, "Cdaq_AO [0-10V] 1":dbl, "Cdaq_AO [0-10V] 2":dbl, "Cdaq_AO [0-10V] 3":dbl}
  T4 = typedef "statoDO_Cdaq.ctl" = cluster{"Scorta 0":bool, "Scorta 1":bool, "Scorta 2":bool, "Scorta 3":bool, "Scorta 4":bool, "Scorta 5":bool, "Scorta 6":bool, "Scorta 7":bool, "Scorta 8":bool, "Scorta 9":bool, "Scorta 10":bool, "Scorta 11":bool, "Scorta 12":bool, "Scorta 13":bool, "Scorta 14":bool, "Scorta 15":bool, "Scorta 16":bool, "Scorta 17":bool, "Scorta 18":bool, "Scorta 19":bool, "Scorta 20":bool, "Scorta 21":bool, "Scorta 22":bool, "Scorta 23":bool, "Scorta 24":bool, "Scorta 25":bool, "Scorta 26":bool, "Scorta 27":bool, "Scorta 28":bool, "Scorta 29":bool, "Scorta 30":bool, "Scorta 31":bool}
  T5 = typedef "MISURE WT.ctl" = cluster{"URMS 1":dbl, "IRMS 1":dbl, "P 1":dbl, "S 1":dbl, "Q 1":dbl, "LAMBDA 1":dbl, "PHI 1":dbl, "F U 1":dbl, "F I 1":dbl, "NONE 1":dbl, "URMS 2":dbl, "IRMS 2":dbl, "P 2":dbl, "S 2":dbl, "Q 2":dbl, "LAMBDA 2":dbl, "PHI 2":dbl, "F U 2":dbl, "F I 2":dbl, "NONE 2":dbl, "URMS 3":dbl, "IRMS 3":dbl, "P 3":dbl, "S 3":dbl, "Q 3":dbl, "LAMBDA 3":dbl, "PHI 3":dbl, "F U 3":dbl, "F I 3":dbl, "NONE 3":dbl, "URMS SIGMA":dbl, "IRMS SIGMA":dbl, "P SIGMA":dbl, "S SIGMA":dbl, "Q SIGMA":dbl, "LAMBDA SIGMA":dbl, "PHI SIGMA":dbl, "F U SIGMA":dbl, "F I SIGMA":dbl, "NONE 4":dbl}
  T6 = typedef "ClusterRes.ctl" = cluster{"Res Ch1":dbl, "Res Ch2":dbl, "Res Ch3":dbl, "Tamb":dbl}
  T7 = typedef "INTERFACCIA.ctl" = cluster{"AI":cluster{"Portate":T8[], "Pressioni":T8[], "Coppie[Nm]":T8[], "Valvole prop %":T8[], "RPM":T8[], "Livelli":T8[], "Temperature":T8[], "Riferimenti %":T8[], "TENSIONI":T8[], "CORRENTI":T8[]}, "DI (logici)":cluster{"Start da pulsantiera":bool, "Stop da pulsantiera":bool, "Reset da pulsantiera":bool, "Sistema OK":bool, "Collaudo abilitato":bool, "Potenza trifase abilitata":bool, "Potenza monofase abilitata":bool, "Potenza DC abilitata":bool, "Potenza DC ECC abilitata":bool, "Start alimentazione AC":bool, "Start alimentazione DC":bool, "Start DC eccitazione":bool, "Teleruttore WT abilitato":bool, "Teleruttore Resistomat abilitato":bool, "Teleruttore corto fasi":bool, "Ramo 1 resistomat":bool, "Ramo 2 resistomat":bool, "Ramo 3 resistomat":bool, "B1 Scelta linea elettrica 1":bool, "B1 Scelta linea elettrica 2":bool, "B1 Scelta linea elettrica 3":bool, "B1 Scelta linea elettrica 4":bool, "B1 Scelta linea elettrica 5":bool, "B2 Scelta linea elettrica 1":bool, "B2 Scelta linea elettrica 2":bool, "B2 Scelta linea elettrica 3":bool, "B2 Scelta linea elettrica 4":bool, "B2 Scelta linea elettrica 5":bool, "Rotore bloccato 1":bool, "Rotore bloccato 2":bool, "FRENO 1 abilitato":bool, "FRENO 1 run":bool, "FRENO 1 senso rotaz":bool, "FRENO 1 ctrl velocità":bool, "FRENO 2 abilitato":bool, "FRENO 2 run":bool, "FRENO 2 senso rotaz":bool, "FRENO 2 ctrl velocità":bool, "ALIM 1 abilitato":bool, "ALIM 1 run":bool, "ALIM 2 abilitato":bool, "ALIM 2 run":bool, "ALIM 3 abilitato":bool, "ALIM 3 run":bool, "FRENO 1 ctrl coppia":bool, "FRENO 2 ctrl coppia":bool, "FRENO 3 ctrl coppia":bool, "DI (logici) aggiuntivi impianto":cluster{"Solo freno abilitato":bool, "Carico resistivo abilitato":bool, "AFE+freno abilitato":bool, "Protezioni chiuse":bool, "Start potenza AFE":bool, "AFE in marcia":bool}, "Misura corrente diretta WT":bool, "Misura corrente sens ext":bool, "Sens ext abilitati":bool}, "AO non scalati":T10, "AO scalati":T10, "DO (logici)":T11}
  T8 = typedef "ClusterMisura_e_Unità_INPUT.ctl" = cluster{"Misura":dbl, "UM":T9, "Descrizione":string}
  T9 = typedef "UnitàMisura.ctl" = enum16{"V", "mA", "Bar", "RPM", "m3/s", "m3/min", "m3/h", "l/s", "l/min", "in3/min", "ft3/min", "gpm", "igpm", "igph", "%", "°C", "m", "Nm", "A"}
  T10 = typedef "Lista AO sistema.ctl" = cluster{"FRENO1 rif vel":dbl, "FRENO1 rif Coppia":dbl, "FRENO2 rif vel":dbl, "FRENO2 rif Coppia":dbl, "ALIM1 rif V":dbl, "ALIM1 rif F":dbl, "ALIM2 rif V":dbl, "ALIM2 rif F":dbl, "ALIM3 rif V":dbl, "ALIM3 rif F":dbl, "Fnom keb":dbl, "Rpm nom keb":dbl, "Pnom keb":dbl, "Inom keb":dbl, "Vnom keb":dbl, "Rpm max keb":dbl, "Tempo rampa keb":dbl, "Tipo Mot keb":dbl, "FRENO  rif Coppia ":dbl, "FRENO  rif  Corrente":dbl}
  T11 = typedef "DOinterfaccia.ctl" = cluster{"Scelta banco 1":bool, "Scelta banco 2":bool, "Scelta banco 3":bool, "FRENO 1 abilita":bool, "FRENO 1 start":bool, "FRENO 1 senso rotaz":bool, "FRENO 1 ctrl velocità":bool, "FRENO 2 abilita":bool, "FRENO 2 start":bool, "FRENO 2 senso rotaz":bool, "FRENO 2 ctrl velocità":bool, "ALIM 1 abilita":bool, "ALIM 1 start":bool, "ALIM 2 abilita":bool, "ALIM 2 start":bool, "ALIM 3 abilita":bool, "ALIM 3 start":bool, "Abilita linea trifase":bool, "Abilita linea monofase":bool, "Abilita linea dc":bool, "Abilita linea dc eccit":bool, "B1 Linea elettrica 1":bool, "B1 Linea elettrica 2":bool, "B1 Linea elettrica 3":bool, "B1 Linea elettrica 4":bool, "B1 Linea elettrica 5":bool, "B2 Linea elettrica 1":bool, "B2 Linea elettrica 2":bool, "B2 Linea elettrica 3":bool, "B2 Linea elettrica 4":bool, "B2 Linea elettrica 5":bool, "Start potenza AC":bool, "Stop pontenza AC":bool, "Start potenza DC":bool, "Stop potenza DC":bool, "Start potenza eccitaz":bool, "Stop potenza eccitaz":bool, "Reset allarmi":bool, "watchdog":bool, "Scala torsiometro B1":bool, "Controllo torsiom B1":bool, "Scala torsiometro B2":bool, "Controllo torsiom B2":bool, "Teleruttore WT abilita":bool, "Teleruttore Resistomat abilita":bool, "Teleruttore corto fasi":bool, "Ramo 1 resistomat":bool, "Ramo 2 resistomat":bool, "Ramo 3 resistomat":bool, "Collaudo in corso":bool, "Allarme presente":bool, "Enable Res Meter":bool, "Bypass Res Meter":bool, "2nd canale Res Meter":bool, "Scala 200/2000 res meter":bool, "Taratura res meter":bool, "FRENO 1 ctrl coppia":bool, "FRENO 2 ctrl coppia":bool, "FRENO 3 ctrl coppia":bool, "Aggiuntivi impianto":cluster{"Senso rotazione alim 1":bool, "Senso rotazione alim 2":bool}, "ALIM 1 stop":bool, "ALIM 2 stop":bool, "ALIM 3 stop":bool, "FRENO 1 stop":bool, "FRENO 2 stop":bool, "FRENO 3 stop":bool, "B1 configurazione freno B":bool, "B2 configurazione freno B":bool, "Abilita scrittura KEB":bool, "Bench Selection (0-B1,1-B2)":bool, "Select current mode":bool, "Select torque mode":bool, "Select speed mode":bool, "Start":bool, "Stop":bool, "Block":bool, "Enable Force mode":bool, "Abilita linea 125 A":bool, "Abilita linea 63 A":bool, "Abilita linea 16 A":bool, "Aum Tensione Variac":bool, "Dim Tesnione Variac":bool, "Abilita ellectro stractura":bool, "Risprinito Emergence":bool, "Abilita collaudo":bool, "Disabilita collaudo":bool, "External Alaram":bool, "Enable external program":bool, "Reset":bool, "Abilita Ingresso Variac":bool, "Abilita Ventilatore Variac":bool, "Abilita Uscita Variac ":bool}
  T12 = typedef "STATO PLC 1.ctl" = cluster{"USCITE PLC":T13, "Stato DI_PLC":cluster{"Sistema OK":bool, "Rotore bloccato":bool, "Scorta 1":bool, "Prova diretto inverter":bool, "Prova con filtro LC":bool, "Teleruttore WT abilitato":bool, "Alim sinus penta abilitato":bool, "Alim sinus penta in marcia":bool, "Freno abilitato":bool, "Freno in marcia":bool, "Senso rotazione freno":bool, "Potenza abilitata":bool, "Scorta 3":bool, "Scorta 4":bool, "scorta 5":bool, "scorta 6":bool}, "AI plc":cluster{"Allarmi 1":dbl, "Allarmi 2":dbl, "Scorta 1":dbl, "Scorta 2":dbl, "RPM mot prova":dbl, "I mot prova":dbl, "RPM freno":dbl, "I freno":dbl, "Scorta 3":dbl, "Scorta 4":dbl}}
  T13 = typedef "Uscite PLC 1.ctl" = cluster{"AO (real) 2":cluster{"SCORTA 1":dbl, "SCORTA 2":dbl, "SCORTA 3":dbl, "SCORTA 4":dbl, "SCORTA 5":dbl, "SCORTA 6":dbl, "SCORTA 7":dbl, "SCORTA 8":dbl}, "statoAO_PLC out":T14, "DO (bit)":T15}
  T14 = typedef "statoAO_plc_1.ctl" = cluster{"Rif Lim coppia freno [%]":dbl, "Rif rpm freno [%]":dbl, "Rif coppia freno [%]":dbl, "Rif V alimentatore [%]":dbl, "Rif F alimentatore [%]":dbl}
  T15 = typedef "StatoDO_PLC_1.ctl" = cluster{"Scelta banco 1":bool, "Set dati motore freno 2":bool, "Diretto inverter":bool, "Filtro LC":bool, "Marcia ALIM (1s)":bool, "Marcia FRENO (1s)":bool, "Stop AFE (1s)":bool, "Stop freno (1s)":bool, "Reset allarmi":bool, "Watchdog":bool, "Senso rotazione":bool, "Abilita collaudo (1s)":bool, "Disabilita collaudo (1s)":bool, "Abilitazione ALIM":bool, "Abilitazione FRENO":bool, "Teleruttore WT":bool, "Senso rot motore prova":bool, "Scorta 7":bool, "Scorta 8":bool, "Scorta 9":bool, "Scorta 10":bool, "Scorta 11":bool, "Scorta 12":bool, "Scorta 13":bool}
  T16 = typedef "Parametri inverter letti.ctl" = cluster{"Menù Misure motore (M000-M030)":cluster{"Rif vel a regime (int)":u16, "Rif vel a regime (dec)":u16, "Rif vel dopo rampe (int)":u16, "Rif vel dopo rampe (dec)":u16, "RPM motore (int)":u16, "RPM motore (dec)":u16, "FREQout inverter":u16, "Rif coppia a regime(Nm)":u16, "Richiesta di coppia (Nm)":u16, "Coppia generata dal motore(Nm)":u16, "Rif coppia a regime(%)":u16, "Richiesta di coppia (%)":u16, "Coppia generata dal motore(%)":u16, "Coppia max richiesta prima delle rampe(Nm)":u16, "Coppia max richiesta dopo le rampe(Nm)":u16, "Limite di velocità prima delle rampe":u16, "Limite di velocità dopo le rampe":u16, "Coppia max richiesta prima delle rampe(%)":u16, "Coppia max richiesta dopo le rampe(%)":u16, "Rif di flusso":u16, "Corrente di uscita":u16, "Capacità termica del motore":u16, "Tensione di uscita":u16, "Potenza di uscita":u16, "Energia consumata (LSword)":u16, "Energia consumata (MSword)":u16, "Tensione bus DC":u16, "Tensione di rete":u16}, "Menù regolatore PID (M018-M024)":cluster{"Rif PID a regime(%)":u16, "Rif pid dopo rampe(%)":u16, "Retroazione del pid(%)":u16, "Errore del pid(%)":u16, "uscita del pid(%)":u16, "Rif del pid dopo le rampe":u16, "Retroazione del pid":u16}, "Menù ingressi digitali (M031-M036)":cluster{"Ingressi digitali ritardati":u16, "Ingressi digitali istantanei":u16, "Moresettiera comando loc":u16, "Morsett comando da seriale":u16, "Morsett comando bus di campo":u16, "Ing dig ausiliari da morsettiera":u16, "Ing dig ausiliari da seriale":u16}, "Menù riferimenti (M037-M051)":cluster{"Rif analog est REF":u16, "Rif analog est AIN1":u16, "Rif analog est AIN2":u16, "Rif analog est XAIN4":u16, "Rif analog est XAIN5":u16, "Rif velocità da seriale(int)":u16, "Rif velocità bus di campo(int)":u16, "Rif coppia da seriale":u16, "Rif coppia bus di campo":u16, "Rif del PID da seriale":u16, "Rif del PID da bus di campo":u16, "Retroazione del PID da seriale":u16, "Retroazione del PIDda bus di campo":u16, "Rif da encoder":u16, "Rif in frequenza":u16, "Rif velocità da seriale(dec)":u16, "Rif velocità bus di campo(dec)":u16}, "Menù rampe (P009-P033)":cluster{"Tempo di dec rampa di vel 1":u16, "Tempo di acc rampa di vel 2":u16, "Tempo di dec rampa di vel 2":u16, "Tempo di acc rampa di vel 1":u16, "Unità di mis tempi rampe vel 1/2":u16, "Tempo di acc rampa di vel 3":u16, "Tempo di dec rampa di vel 3":u16, "Tempo di acc rampa di vel 4":u16, "Tempo di dec rampa di vel 4":u16, "Unità di mis tempi rampe vel 3/4":u16, "Selettore arrottondam rampe":u16, "Tempo di arrotond iniz rampa acc":u16, "Tempo di arrotond finale rampa acc":u16, "Tempo di arrotond iniz rampa dec":u16, "Tempo di rampa di salita rif coppia":u16, "Tempo di rampa di discesa rif coppia":u16, "Unità di misura rampa coppia":u16, "Tempo rampa acc marcia jog":u16, "Tempo rampa dec marcia jog":u16, "Reset acc ai cambi pendenza":u16, "rampa di acc in fire mode":u16, "rampa di dec in fire mode":u16, "Tempo di arrotond finale rampa dec":u16}, "Menù controllo motore(C008-C128)":cluster{"Numero motori configurati":u16, "Tipo algoritmo di controllo Mot1":u16, "Tipo rif Mot1":u16, "Tensione nominale rete":u16, "Retroaz di vel da encoder Mot1":u16, "Tipo curva V/f Mot1":u16, "Rotazione delle fasi Mot1":u16, "Freq nominale del motore Mot1":u16, "RPM nominali del motore Mot1":u16, "Potenza nominale del motore Mot1":u16, "Corrente nominale del motore Mot1":u16, "Tensione nominale del motore mot1":u16, "Potenza a vuoto del motore Mot1":u16, "Corrente a vuoto del motore Mot1":u16, "Resistenza statorica del motore Mot1":u16, "Induttanza di dispersione Mot1":u16, "Induttanza mutua motore":u16, "Costante di tempo rotorica":u16, "Costante di tempo filtro pb":u16, "Velocità minima motore":u16, "Velocità massima motore":u16}, "Menù configurazione PID":cluster{"Selezione riferimento n.1":u16, "Selezione retroazione n.1":u16, "Modalità di fuzionamento PID":u16, "Termine derivativo calcolato su err o mis":u16, "Proporz moltiplica deriv e integrale":u16, "Azione del PID":u16}, "ID":dbl, "Menù uscite digitali":cluster{"MDO4 Inverter pronto":u16}, "Fcarrier":cluster{"Fcarrier Min (Hz)":u16, "Fcarrier Max (Hz)":u16}, "stato inverter M089":dbl, "Riferimenti":cluster{"Rif tensione":u16, "Rif velocità":u16}, "Comunicazione":bool, "Modalità stop":dbl}
  T17 = typedef "STATO PLC 2.ctl" = cluster{"USCITE PLC":T18, "Stato DI_PLC":cluster{"Sistema ok":bool, "Relè Resistomat abilitato":bool, "Freno abilitato":bool, "Freno in marcia":bool, "scorta b":bool, "scorta a":bool, "scorta 1":bool, "scorta 2":bool, "scorta 3":bool, "scorta 4":bool, "Scorta 5":bool, "Scorta 6":bool, "Scorta 7":bool, "Scorta 8":bool, "Scorta 9":bool, "Scorta 10":bool}, "AI plc":cluster{"Allarmi 1":dbl, "Allarmi 2":dbl, "TC 1":dbl, "TC 2":dbl, "TC 3":dbl, "TC 4":dbl, "TC 5":dbl, "TC 6":dbl, "TC 7":dbl, "TC 8":dbl, "PT1000 1":dbl, "PT1000 2":dbl, "PT1000 3":dbl, "PT1000 4":dbl}}
  T18 = typedef "Uscite PLC 2.ctl" = cluster{"AO (real) 2":cluster{"SCORTA 1":dbl, "SCORTA 2":dbl, "SCORTA 3":dbl, "SCORTA 4":dbl, "SCORTA 5":dbl, "SCORTA 6":dbl, "SCORTA 7":dbl, "SCORTA 8":dbl}, "statoAO_PLC out":T19, "DO (bit)":T20}
  T19 = typedef "statoAO_plc_2.ctl" = cluster{"Condensatori":dbl, "Scorta 1":dbl, "Scorta 2":dbl}
  T20 = typedef "StatoDO_PLC_2.ctl" = cluster{"Relè misura resistomat":bool, "Misura res ramo 1":bool, "Misura res ramo 2":bool, "Misura res ramo 3":bool, "Scelta banco 2":bool, "Scala Torsiometro":bool, "Ctrl torsiometro":bool, "Select current mode":bool, "Select Torque mode":bool, "Select speed mode":bool, "Watchdog":bool, "Scorta":bool, "Scorta 2":bool, "Scorta 3":bool, "Scorta 4":bool, "Scorta 5":bool, "Bench selection":bool, "External alarm":bool, "Enable external program":bool, "Reset allarmi":bool, "Start":bool, "Stop":bool, "Block":bool, "Scorta 6":bool}
  T21 = typedef "STATO PLC 3.ctl" = cluster{"USCITE PLC":T22, "Stato DI_PLC":cluster{"Sistema OK":bool, "Rotore bloccato":bool, "Filtro LC":bool, "Bypass Filtro LC":bool, "Scelta Trasformatore":bool, "Scelta Bypass trasformatore":bool, "Teleruttore wt abilitato":bool, "Alimentatore abilitato":bool, "Alimentatore in marcia":bool, "Scorta 1":bool, "Scorta 2":bool, "Scorta 3":bool, "Potenza abilitata":bool, "Alimentatore in allarme":bool, "Scorta 4":bool, "Conferma dati KEB":bool, "Scorta 5":bool, "Warning Inverter Alimentatore":bool, "Variac Abilitato":bool, "Linea 125 A abilitata":bool, "Linea 63 A abilitata":bool, "Linea 16 A abilitata":bool, "Scorta 6":bool, "Enable force mode":bool}, "AI plc":cluster{"Allarmi 1":dbl, "Allarmi 2":dbl, "RPM motore prova":dbl, "Corrente motore prova":dbl, "RPM freno":dbl, "Corrente freno":dbl, "Tipo motore keb":dbl, "I nom keb":dbl, "RPM nom keb":dbl, "V nom keb":dbl, "F nom keb":dbl, "T rampa keb":dbl, "scorta":dbl, "Scorta 2":dbl}}
  T22 = typedef "Uscite PLC 3.ctl" = cluster{"AO (real) 2":cluster{"SCORTA 1":dbl, "SCORTA 2":dbl, "SCORTA 3":dbl, "SCORTA 4":dbl, "SCORTA 5":dbl, "SCORTA 6":dbl, "SCORTA 7":dbl, "SCORTA 8":dbl}, "statoAO_PLC out":T23, "DO (bit)":T24}
  T23 = typedef "statoAO_plc_3.ctl" = cluster{"Rif velocità alimentatore":dbl, "Scorta":dbl, "Tipo Motore  keb":dbl, "I nom keb":dbl, "RPM nom keb":dbl, "V nom keb":dbl, "F nom keb":dbl, "t rampa keb":dbl}
  T24 = typedef "StatoDO_PLC_3.ctl" = cluster{"Select linea Inverter":bool, "Abilita sense wattmetro":bool, "Bypass filtro LC":bool, "Filtro LC":bool, "Bypass trasformatore":bool, "Trasformatore":bool, "Abilita uscite variac":bool, "Abilita linea 125 A":bool, "Abilita linea 63 A":bool, "Abilita linea 16 A":bool, "Abilita Scrittura Dati Keb":bool, "Abilita alimentatore":bool, "Marcia alimentatore (1s)":bool, "Stop alimentatore (1s)":bool, "Senso rot mot prova":bool, "Watchdog":bool, "Aumenta tensione variac":bool, "Diminuisci tensione variac ":bool, "Blocco elettroserrature":bool, "Ripristino emergence":bool, "Abilita ingresso variac":bool, "Abilita ventilatore variac":bool, "Reset Allarm":bool, "Scorta 1":bool, "Scorta 2":bool, "Scorta 3":bool, "Scorta 4":bool, "Scorta 5":bool, "Scorta 6":bool, "Scorta 7":bool, "Scorta 8":bool, "Scorta 9":bool, "Abilita collaudo":bool, "Disabilita collaudo ":bool, "Scorta 10":bool, "Scorta 11":bool, "Scorta 12":bool, "Scorta 13":bool, "Scorta 14":bool, "Scorta 15":bool}
  T25 = typedef "Parametri DCREG letti.ctl" = cluster{"Parametri di misura":cluster{"M000":dbl, "M001":dbl, "M002":dbl, "M003":dbl, "M004":dbl, "M005":dbl, "M006":dbl, "M007":dbl, "M008":dbl, "M009":dbl, "M010":dbl, "M011":dbl, "M012":dbl, "M013":dbl, "M014":dbl, "M015":dbl, "M016":dbl, "M017":dbl, "M018":dbl, "M019":dbl, "M020":dbl, "M021":dbl, "M022":dbl, "M023":dbl, "M024":dbl, "M025":dbl, "M026":dbl, "M027":dbl, "M028":dbl, "M029":dbl, "M030":dbl, "M031":dbl}, "Parametri di programmazione":cluster{"P000":dbl, "P001":dbl, "P002":dbl, "P003":dbl, "P004":dbl, "P005":dbl, "P006":dbl, "P010":dbl, "P011":dbl, "P012":dbl, "P013":dbl, "P014":dbl, "P015":dbl, "P016":dbl, "P030":dbl, "P031":dbl, "P032":dbl, "P033":dbl, "P034":dbl, "P035":dbl, "P036":dbl, "P037":dbl, "P038":dbl, "P039":dbl, "P040":dbl, "P050":dbl, "P051":dbl, "P052":dbl, "P053":dbl, "P054":dbl, "P055":dbl, "P056":dbl, "P057":dbl, "P058":dbl, "P059":dbl, "P060":dbl, "P061":dbl, "P062":dbl, "P070":dbl, "P071":dbl, "P073":dbl, "P074":dbl, "P076":dbl, "P077":dbl, "P079":dbl, "P080":dbl, "P082":dbl, "P083":dbl, "P084":dbl, "P085":dbl, "P086":dbl, "P087":dbl, "P088":dbl, "P100":dbl, "P101":dbl, "P102":dbl, "P103":dbl, "P104":dbl, "P110":dbl, "P111":dbl, "P120":dbl, "P121":dbl, "P122":dbl, "P123":dbl, "P124":dbl, "P125":dbl, "P126":dbl, "P127":dbl, "P128":dbl, "P129":dbl, "P130":dbl, "P131":dbl, "P132":dbl, "P133":dbl, "P134":dbl, "P150":dbl, "P151":dbl, "P152":dbl, "P153":dbl, "P154":dbl, "P155":dbl, "P156":dbl, "P157":dbl, "P158":dbl, "P170":dbl, "P171":dbl, "P172":dbl, "P173":dbl, "P174":dbl, "P175":dbl, "P176":dbl, "P177":dbl, "P178":dbl, "P179":dbl, "P180":dbl, "P181":dbl, "P182":dbl, "P183":dbl, "P184":dbl, "P185":dbl, "P186":dbl, "P187":dbl, "P188":dbl, "P189":dbl, "P190":dbl, "P191":dbl, "P192":dbl, "P193":dbl, "P194":dbl, "P195":dbl, "P196":dbl, "P197":dbl, "P198":dbl, "P199":dbl, "P211":dbl, "P212":dbl, "P213":dbl, "P214":dbl, "P215":dbl, "P216":dbl, "P217":dbl, "P221":dbl, "P222":dbl, "P223":dbl, "P224":dbl, "P230":dbl, "P231":dbl, "P240":dbl, "P250":dbl, "P251":dbl}, "Parametri di configurazione":cluster{"C000":dbl, "C001":dbl, "C002":dbl, "C010":dbl, "C011":dbl, "C012":dbl, "C014":dbl, "C015":dbl, "C016":dbl, "C017":dbl, "C018":dbl, "C030":dbl, "C050":dbl, "C051":dbl, "C052":dbl, "C060":dbl, "C061":dbl, "C062":dbl, "C063":dbl, "C070":dbl, "C072":dbl, "C074":dbl, "C090":dbl, "C091":dbl, "C092":dbl, "C093":dbl, "C094":dbl, "C100":dbl, "C101":dbl, "C102":dbl, "C103":dbl, "C105":dbl, "C106":dbl, "C107":dbl, "C108":dbl, "C110":dbl, "C111":dbl, "C112":dbl, "C120":dbl, "C121":dbl, "C122":dbl, "C130":dbl, "C131":dbl, "C132":dbl, "C133":dbl, "C134":dbl, "C135":dbl, "C141":dbl, "C142":dbl, "C143":dbl, "C150":dbl, "C151":dbl, "C153":dbl, "C154":dbl, "C155":dbl, "C156":dbl, "C157":dbl, "C158":dbl, "C159":dbl, "C160":dbl, "C161":dbl, "C162":dbl, "C163":dbl, "C164":dbl, "C165":dbl, "C170":dbl}, "Codice allarme":dbl, "Comunicazione":bool}
  T26 = typedef "Cluster INFO.ctl" = cluster{"Scelta wattmetro":cluster{"Wattmetro":T27}, "SET RPM":dbl, "SET TEMP":dbl, "Array banchi":T28[], "Array valvole linee avvio/fermata":cluster{"Valvole avvio":cluster{"Set valvole avvio?":bool, "% valvole avvio":dbl[]}, "Valvole fermata":cluster{"Set valvole fermata?":bool, "% valvole fermata":dbl[]}}[], "banco selezionato":i8, "Nomi valvole prop sistema":string[], "canale-- sensore":string[][], "Attriti B1":dbl[][], "Attriti B2":dbl[][], "Collegamento elettrico":cluster{"ALIMENTAZIONE ELETTRICA":T29, "ID":i16, "#rami freddo\\eq term resmeter":i16, "#rami riscaldamento resmeter":i16, "#rami freddo\\eq term resistomat":i16, "#rami riscaldamento resistomat":i16, "CALCOLI":T30}, "lingua":i16, "Costanti collaudo":cluster{"P [bar]":dbl, "T amb. [°C]":dbl, "Umidità [%]":dbl, "T acqua [°C] 2":dbl}, "OPZIONI MISURE RES":cluster{"MISURA A FREDDO":enum16{"NESSUNO", "RESISTOMAT", "RES METER", "ENTRAMBI"}, "MISURA EQ. TERMICO":enum16{"NESSUNO", "RESISTOMAT", "RES METER", "ENTRAMBI"}, "MISURA DT PROVA IN CORSO":enum16{"NESSUNO", "RESISTOMAT - CON FERMATE", "RES METER - CON FERMATE", "RES METER - CONTINUO"}, "MISURE PRIMA E DOPO":enum16{"NESSUNO", "RESISTOMAT", "RES METER"}, "STRUMENTI PRESENTI":enum16{"NESSUNO", "RESISTOMAT", "RES METER", "ENTRAMBI"}}, "Dati targa motore":cluster{"Vnom":dbl, "Fnom":dbl, "Inom":dbl, "Cnom":dbl, "Npoli":dbl, "Scorta 1":dbl, "Scorta 2":dbl, "Scorta 3":dbl}}
  T27 = typedef "WT SELECTION.ctl" = enum32{"No Selection", "WT230", "WT333", "WT1800", "WT330", "VIW", "APLUS"}
  T28 = typedef "Definizione linea.ctl" = cluster{"Nome":string, "Tors. scala1":i32, "Tors. scala2":i32, "rpm":i32, "TAMB":i32, "Indici Temperature":i16[], "Indice freno":i16, "alimentatore trifase":i16, "alimentatore monofase":i16, "alimentatore dc arm":i16, "alimentatore dc ecc":i16, "alimentatore dc mp":i16}
  T29 = typedef "Collegamenti_elettrici.ctl" = enum16{"AC TRIFASE", "AC TRIFASE + FRENO", "AC MONOFASE", "DC CON ECCITAZIONE", "DC CON ECCITAZIONE + FRENO", "DC NO ECCITAZIONE", "DC NO ECCITAZIONE + FRENO", "FRENO TRASC + AFE", "SOLO FRENO", "CARICO RESISTIVO", "GENERICO", "SOLO ACQUISITORE", "SCORTA 4", "SCORTA 5", "SCORTA 6"}
  T30 = typedef "Control Calcoli.ctl" = enum16{"AC TRIFASE", "AC MONOFASE", "DC ECCITAZIONE", "DC NO ECCITAZIONE", "POMPA TRIFASE", "POMPA MONOFASE", "GENERICO", "TRASFORMATORE", "ALTERNATORE TRASCINATO", "GRUPPO ELETTROGENO"}
  T31 = typedef "MISURE NM.ctl" = cluster{"Banco":string, "Anno":string, "Numero":string, "Ntabella":string, "Misura":string, "Tipo Prova":string, "ProgressivoAcq":string, "Descrizione":string, "Data_ora":string, "t. acq [h:m:s]":string, "t. acq [min]":string, "t. acq [s]":string, "n [rpm]":string, "f [Hz]":string, "U1[V]":string, "U2 [V]":string, "U3 [V]":string, "U123_media [V]":string, "I1[A]":string, "I2[A]":string, "I3[A]":string, "I123_media [A]*I":string, "I_123_sbil [%]":string, "Ulin[V]":string, "Uc [V]":string, "Uaux [V]":string, "Ilin[A]*I":string, "Imar[A]":string, "Iaux[A]":string, "Uarm[V]":string, "Uecc[V]":string, "Iarm[A]*I":string, "Iecc[A]":string, "pf":string, "P1 [W]":string, "P1 [kW]":string, "Q [VAR]":string, "Q [kVAR]":string, "S [VA]":string, "S [kVA]":string, "P1arm[W]":string, "P1ecc[W]":string, "Parm[kW]":string, "P1ecc[kW]":string, "Cond[uF]":string, "P1_linea_6fili[W]":string, "P1_linea_6fili[kW]":string, "eta_gr_6fili [%]":string, "eta_inverter_6fili [%]":string, "pf_linea_6fili":string, "U4 [V]":string, "U5 [V]":string, "U6 [V]":string, "U456_media [V]":string, "I4 [A]":string, "I5 [A]":string, "I6 [A]":string, "I456_media [A]":string, "C [Nm]*C":string, "Cric [Nm]":string, "Cric\\Cnom":string, "Iric[A]":string, "Iric\\Inom":string, "P2_mecc [W]":string, "P2_mecc [kW]":string, "eta motore [%]":string, "Scorr[%]":string, "Tamb[°C]":string, "R1[ohm]":string, "R2[ohm]":string, "R3[ohm]":string, "Rmedia[ohm]":string, "DT_R1[°C]":string, "DT_R2[°C]":string, "DT_R3[°C]":string, "DT_media[°C]":string, "R_marcia[ohm]":string, "R_aux[ohm]":string, "DT_marcia[°C]":string, "DT_aux[°C]":string, "R_Arm[ohm]":string, "R_Ecc[ohm]":string, "DT_Arm[°C]":string, "DT_Ecc[°C]":string, "TambFreddo[°C]":string, "R1_freddo[ohm]":string, "R2_freddo[ohm]":string, "R3_freddo[ohm]":string, "Rmedia_freddo[ohm]":string, "R_Marcia_freddo[ohm]":string, "R_Aux_freddo[ohm]":string, "R_Arm_freddo[ohm]":string, "R_Ecc_freddo[ohm]":string, "TC1 [°C]":string, "TC2 [°C]":string, "TC3 [°C]":string, "TC4 [°C]":string, "TC5 [°C]":string, "TC6 [°C]":string, "TC7 [°C]":string, "TC8 [°C]":string, "PT1000_1[°C]":string, "PT1000_2[°C]":string, "PT1000_3[°C]":string, "Vdc eccitatrice[V]":string, "Idc eccitatrice[A]":string, "Vdc rotore[V]":string, "Idc rotore[A]":string, "Vac rotore[V]":string, "Iac rotore[V]":string, "V dinamo[V]":string, "Portata Q":string, "Pressione H":string, "U1'[V]":string, "U2'[V]":string, "U3'[V]":string, "I1'[A]":string, "I2'[A]":string, "I3'[A]":string, "U''R-N":string, "U''S-N":string, "U'' T-N":string, "U''R-S":string, "U''R-T":string, "U''S-T":string, "I1''[A]":string, "I2''[A]":string, "I3''[A]":string, "F''[Hz]":string, "P''[kW]":string, "CosFi''":string, "PT1000_4[°C]":string, "Scorta 3":string}
  T32 = enum16{"NESSUNO", "RESISTOMAT - CON FERMATE", "RES METER - CON FERMATE", "RES METER - CONTINUO"}
  T33 = cluster{"ALIMENTAZIONE ELETTRICA":T29, "ID":i16, "#rami freddo\\eq term resmeter":i16, "#rami riscaldamento resmeter":i16, "#rami freddo\\eq term resistomat":i16, "#rami riscaldamento resistomat":i16, "CALCOLI":T30}
  T34 = cluster{"MISURA A FREDDO":enum16{"NESSUNO", "RESISTOMAT", "RES METER", "ENTRAMBI"}, "MISURA EQ. TERMICO":enum16{"NESSUNO", "RESISTOMAT", "RES METER", "ENTRAMBI"}, "MISURA DT PROVA IN CORSO":enum16{"NESSUNO", "RESISTOMAT - CON FERMATE", "RES METER - CON FERMATE", "RES METER - CONTINUO"}, "MISURE PRIMA E DOPO":enum16{"NESSUNO", "RESISTOMAT", "RES METER"}, "STRUMENTI PRESENTI":enum16{"NESSUNO", "RESISTOMAT", "RES METER", "ENTRAMBI"}}
  T35 = cluster{"Dt media":dbl, "Res media":dbl, "Res freddo media":dbl}
  T36 = cluster{"I1 [A]":dbl, "I2 [A]":dbl, "I3 [A]":dbl}
  T37 = cluster{"ECCITATRICE":cluster{"VDC [V]":dbl, "IDC [A]":dbl}, "ROTORE":cluster{"Vdc [V]":dbl, "Idc [A]":dbl, "Vac [V]":dbl, "Iac [A]":dbl}}
  T38 = cluster{"U1 [V]":dbl, "U2 [V]":dbl, "U3 [V]":dbl, "I1 [A]":dbl, "I2 [A]":dbl, "I3 [A]":dbl}
  T39 = cluster{"Tensione [V]":dbl, "Corrente [A]":dbl, "Frequenza [Hz]":dbl, "Velocità [RPM]":dbl, "I saldatura [A]":dbl}
  T40 = cluster{"Q":dbl, "H":dbl, "U1 [V]":dbl, "U2 [V]":dbl, "U3 [V]":dbl, "I1 [A]":dbl, "I2 [A]":dbl, "I3 [A]":dbl}
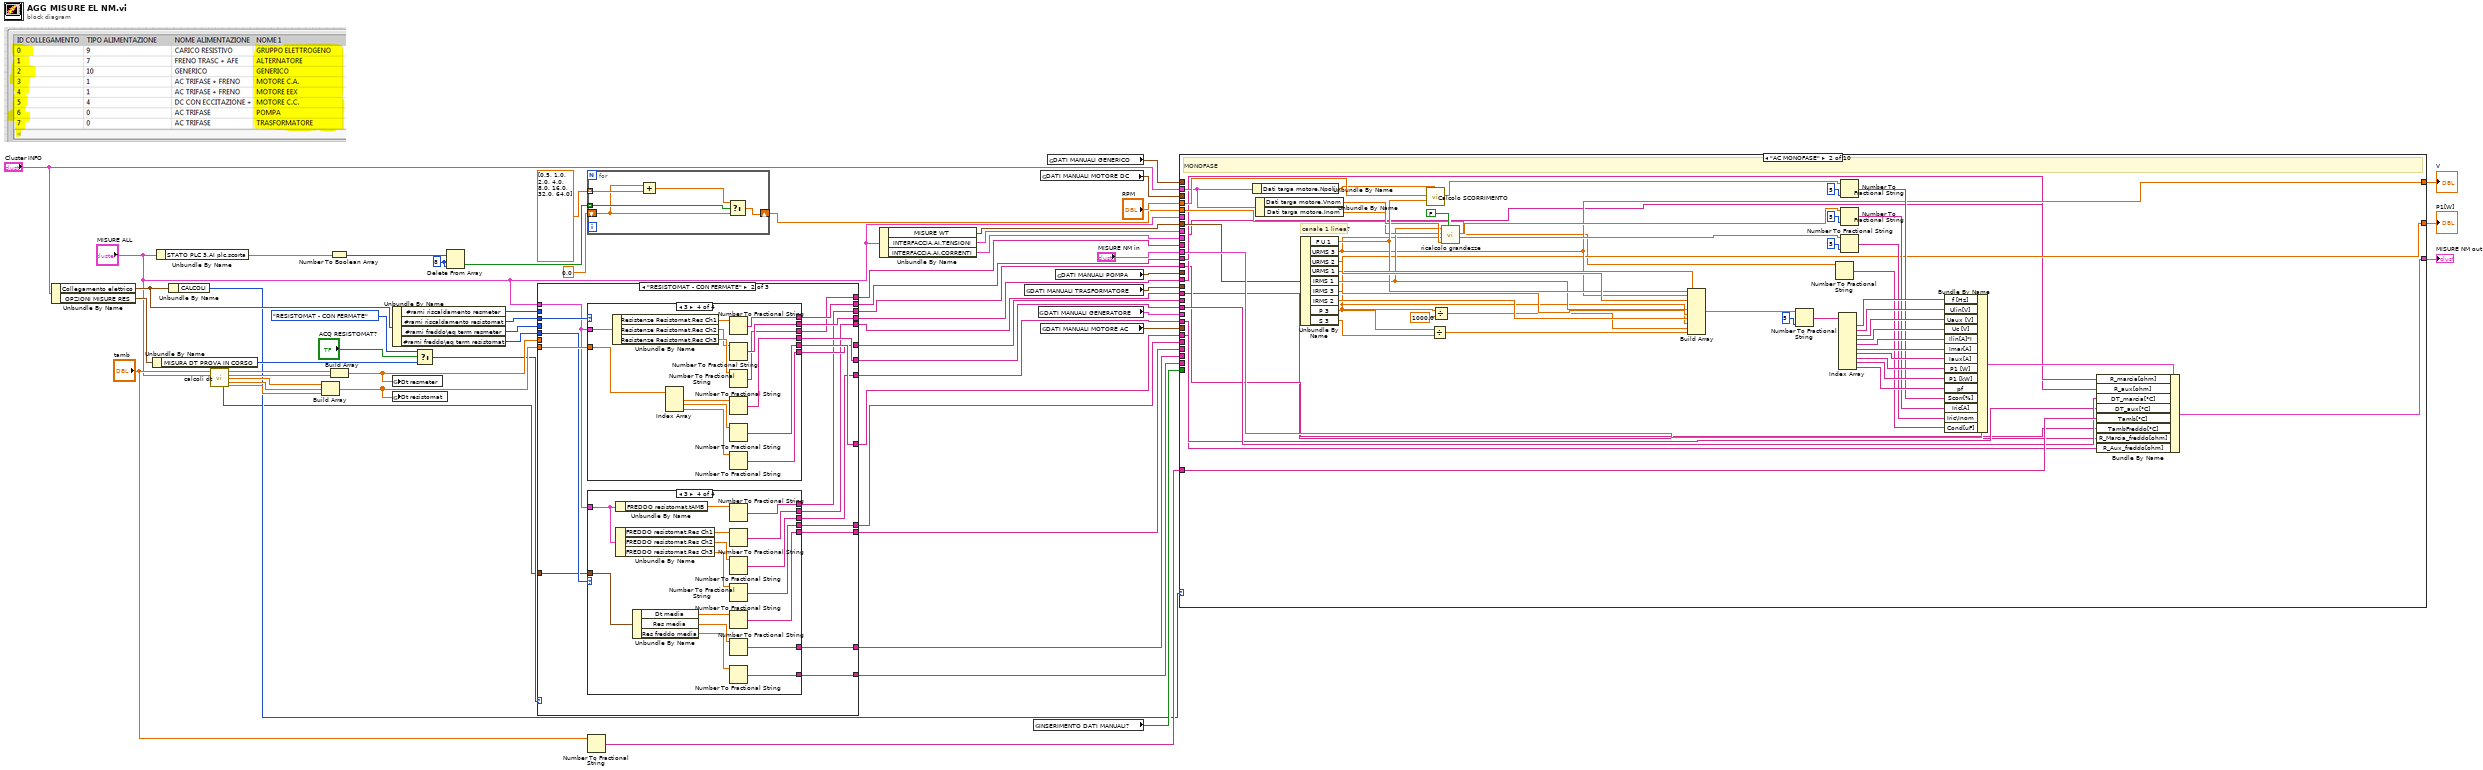
[diagram p0: block diagram]
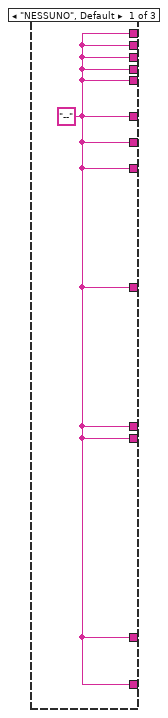
[diagram p2: hidden frame]
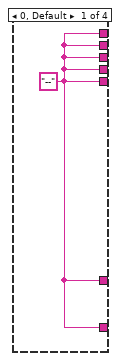
[diagram p3: hidden frame]
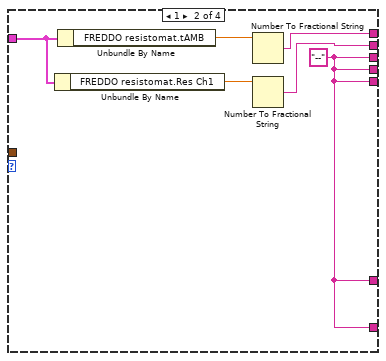
[diagram p4: hidden frame]
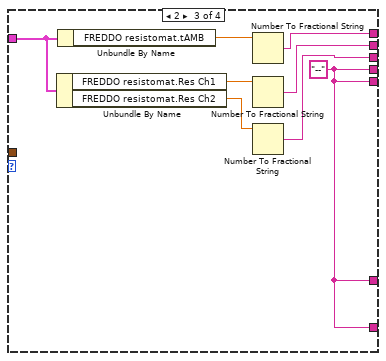
[diagram p5: hidden frame]
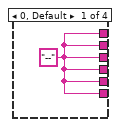
[diagram p6: hidden frame]
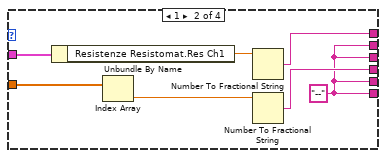
[diagram p7: hidden frame]
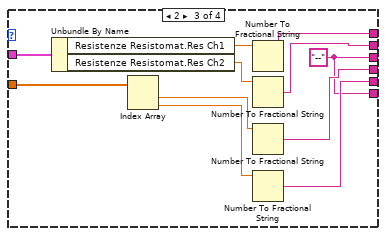
[diagram p8: hidden frame]
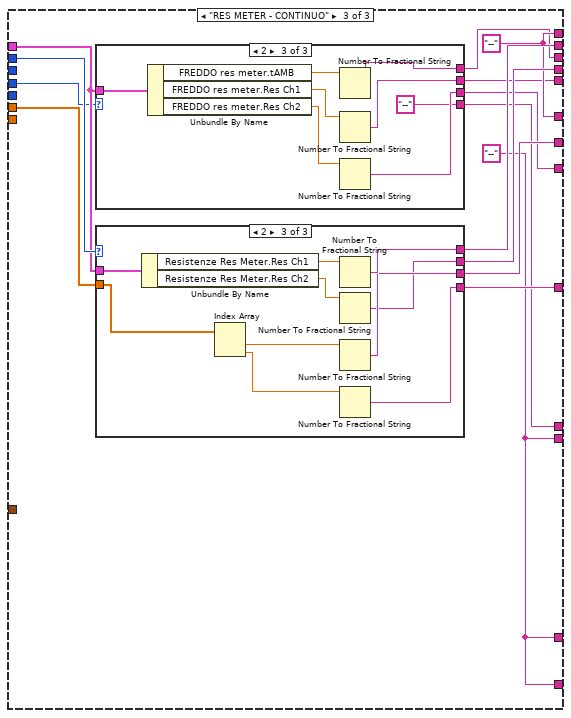
[diagram p9: hidden frame]
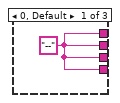
[diagram p10: hidden frame]
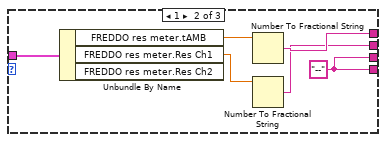
[diagram p11: hidden frame]
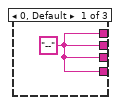
[diagram p12: hidden frame]
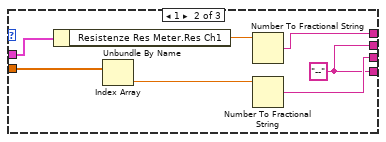
[diagram p13: hidden frame]
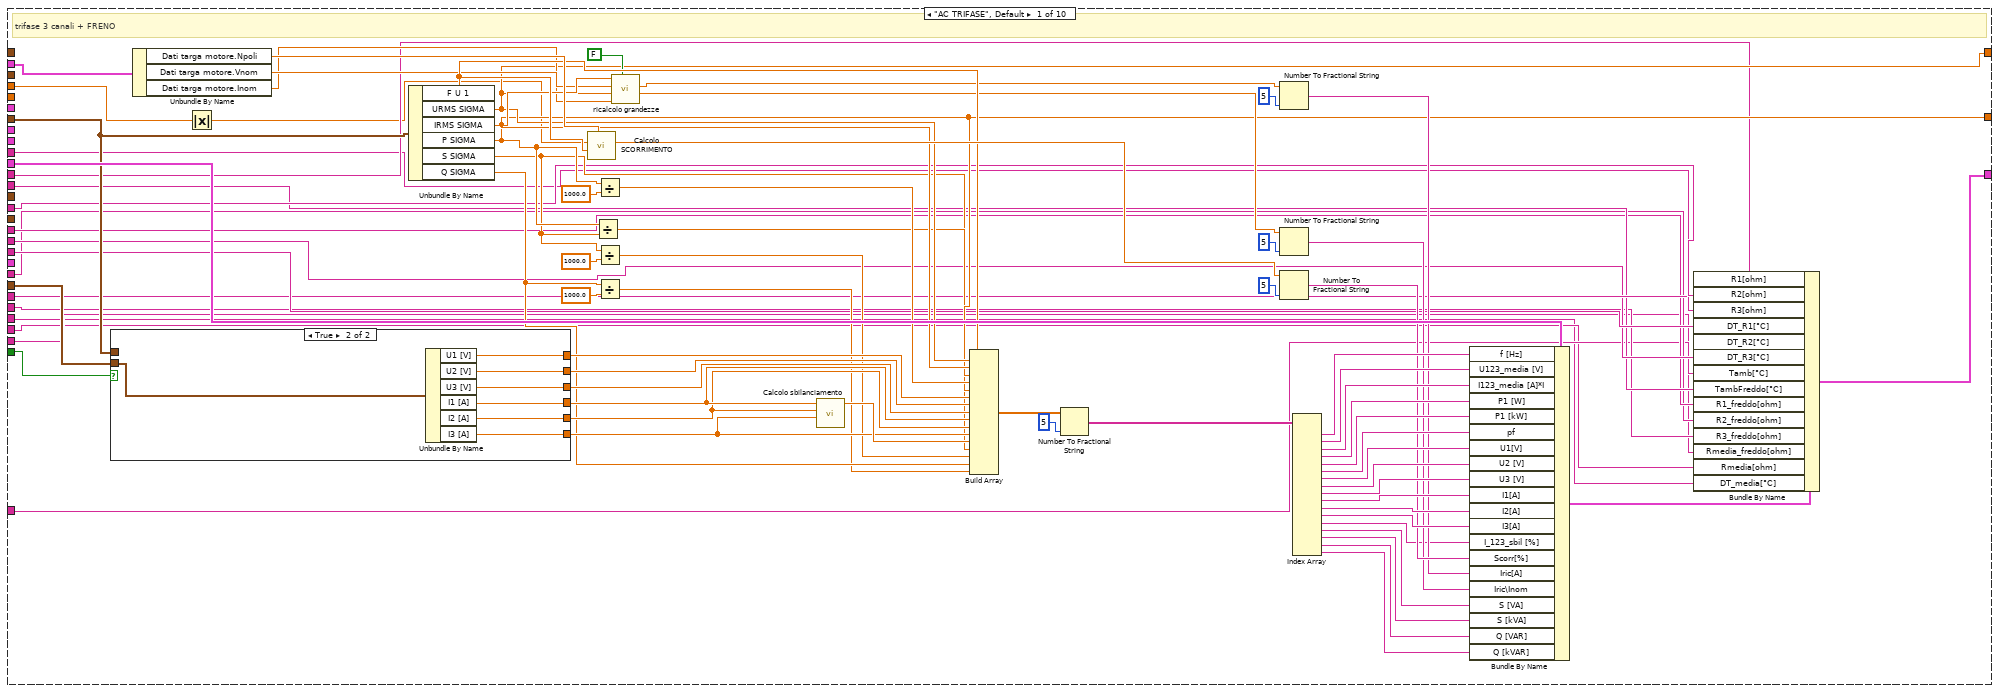
[diagram p14: hidden frame]
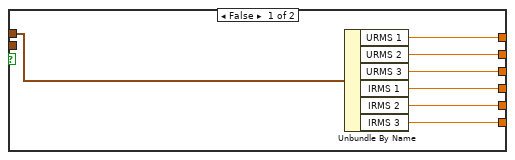
[diagram p15: hidden frame]
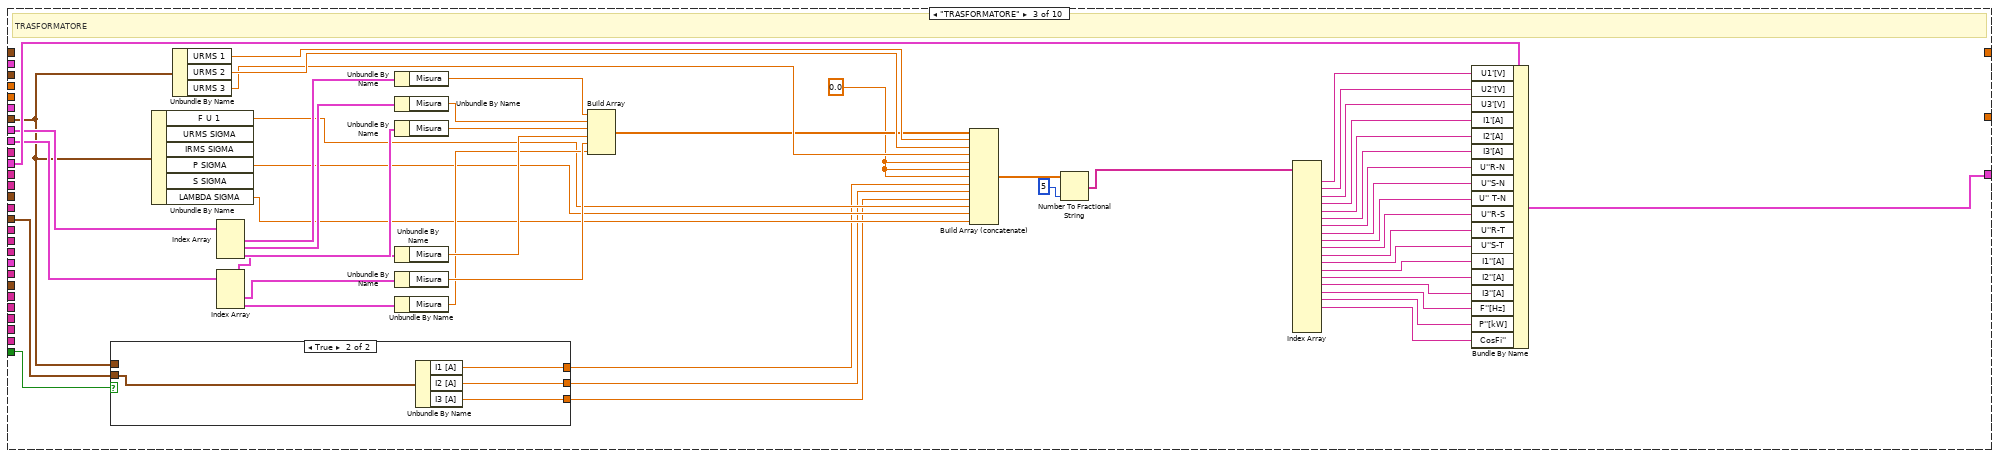
[diagram p16: hidden frame]
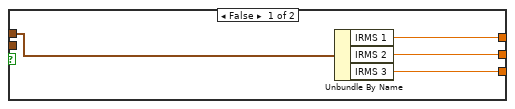
[diagram p17: hidden frame]
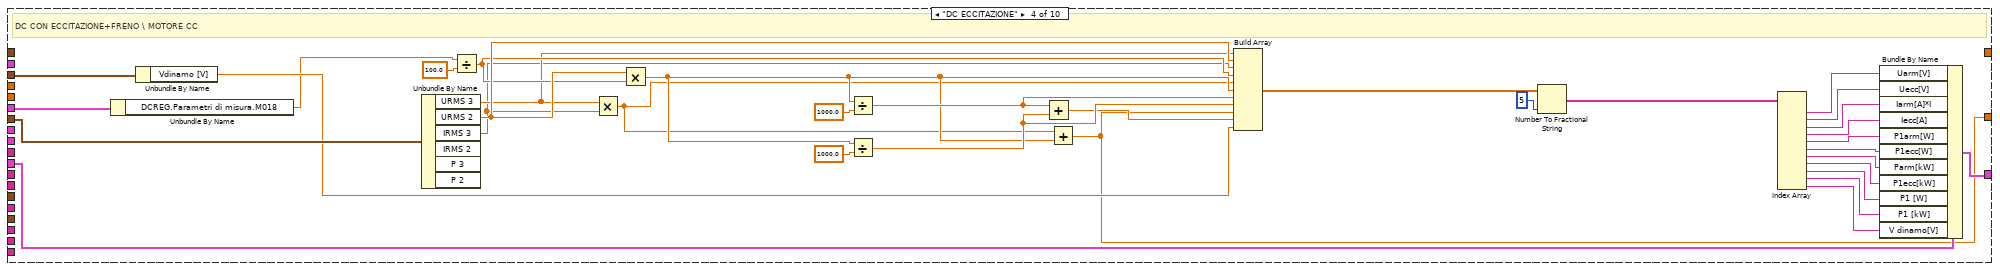
[diagram p18: hidden frame]
diagram:
  w41 = 8 ("index")
  n1 = Unbundle By Name("Cluster INFO") -> ("Collegamento elettrico"=w28:T33, "OPZIONI MISURE RES"=w27:T34)
  n2 = Unbundle By Name(w27) -> ("MISURA DT PROVA IN CORSO"=w9:T32)
  n3 = Unbundle By Name("MISURE ALL") -> ("STATO PLC 3.AI plc.scorta"=w46:dbl)
  n4 = Unbundle By Name(w28) -> ("CALCOLI"=w5:T30)
  n5 = call "calcoli dt.vi"("tamb"="tamb", "MISURE ALL"="MISURE ALL") -> ("Dt resMeter CH1"=w54:dbl, "Dt resMeter CH2"=w53:dbl, "Dt resistomat CH1"=w31:dbl, "Dt resistomat CH2"=w52:dbl, "res medie"=w4:T35, "Dt resistomat CH3"=w51:dbl)  [unwired: 8 in]
  n6 = Build Array(w31, w52, w51) -> (w25:dbl[])
  n7 = Build Array(w54, w53) -> (w16:dbl[])
  n8 = Number To Boolean Array(number=w46) -> (Boolean array=w44:bool[])
  n9 = Unbundle By Name(w28) -> ("#rami riscaldamento resmeter"=w17:i16, "#rami riscaldamento resistomat"=w24:i16, "#rami freddo\\eq term resmeter"=w10:i16, "#rami freddo\\eq term resistomat"=w15:i16)
  n10 = global write "Global DT per visualizzazione.vi" "Dt resmeter"(w16) -> ()
  n11 = global write "Global DT per visualizzazione.vi" "Dt resistomat"(w25) -> ()
  n12 = Select(t=T32."RESISTOMAT - CON FERMATE", s="ACQ RESISTOMAT?", f=w9) -> (s? t:f=w7:T32)
  n13 = Delete From Array(array=w44, length=w41, index=w41) -> (deleted portion=w43:bool[])  [unwired: 1 out]
  n14 = case shown="\"RESISTOMAT - CON FERMATE\"" w7 {
    tunnel: "MISURE ALL" -> [_ w69 w148]
    tunnel: w25 -> [_ w76 _]
    tunnel: w24 -> [_ w77 _]
    tunnel: [w59 w75 w153] -> w23
    tunnel: [w59 w74 w151] -> w22
    tunnel: [w59 w73 w149] -> w21
    tunnel: [w59 w72 w152] -> w20
    tunnel: [w59 w71 w150] -> w19
    tunnel: [w59 w70 w149] -> w18
    tunnel: w17 -> [_ _ w155]
    tunnel: w16 -> [_ _ w154]
    tunnel: w15 -> [_ w68 _]
    tunnel: [w59 w67 w145] -> w14
    tunnel: [w59 w66 w144] -> w13
    tunnel: [w59 w65 w143] -> w12
    tunnel: [w59 w64 w146] -> w11
    tunnel: w10 -> [_ _ w147]
    tunnel: w4 -> [_ w63 _]
    tunnel: [w59 w62 w142] -> w1
    tunnel: [w59 w61 w142] -> w2
    tunnel: [w59 w60 w142] -> w3
    frame "NESSUNO", Default {
      w59 = "--"
    }
    frame "RESISTOMAT - CON FERMATE" {
      n15 = case shown="3" w77 {
        tunnel: w69 -> [_ w116 w127 w141]
        tunnel: w76 -> [_ w115 w126 w140]
        tunnel: [w109 w112 w121 w133] -> w75
        tunnel: [w109 w111 w120 w130] -> w72
        tunnel: [w109 w110 w119 w132] -> w74
        tunnel: [w109 w110 w118 w129] -> w71
        tunnel: [w109 w110 w117 w131] -> w73
        tunnel: [w109 w110 w117 w128] -> w70
        frame 0, Default {
          w109 = "--"
        }
        frame 1 {
          w110 = "--"
          n16 = Unbundle By Name(w116) -> ("Resistenze Resistomat.Res Ch1"=w114:dbl)
          n17 = Index Array(array=w115) -> (element=w113:dbl)  [unwired: 1 in]
          n18 = Number To Fractional String(number=w114) -> (F-format string=w112:string)  [unwired: 3 in]
          n19 = Number To Fractional String(number=w113) -> (F-format string=w111:string)  [unwired: 3 in]
        }
        frame 2 {
          w117 = "--"
          n20 = Unbundle By Name(w127) -> ("Resistenze Resistomat.Res Ch1"=w125:dbl, "Resistenze Resistomat.Res Ch2"=w124:dbl)
          n21 = Index Array(array=w126) -> (element #1=w123:dbl, element #2=w122:dbl)  [unwired: 2 in]
          n22 = Number To Fractional String(number=w125) -> (F-format string=w121:string)  [unwired: 3 in]
          n23 = Number To Fractional String(number=w124) -> (F-format string=w119:string)  [unwired: 3 in]
          n24 = Number To Fractional String(number=w123) -> (F-format string=w120:string)  [unwired: 3 in]
          n25 = Number To Fractional String(number=w122) -> (F-format string=w118:string)  [unwired: 3 in]
        }
        frame 3 {
          n26 = Unbundle By Name(w141) -> ("Resistenze Resistomat.Res Ch1"=w139:dbl, "Resistenze Resistomat.Res Ch2"=w137:dbl, "Resistenze Resistomat.Res Ch3"=w138:dbl)
          n27 = Index Array(array=w140) -> (element #1=w136:dbl, element #2=w135:dbl, element #3=w134:dbl)  [unwired: 3 in]
          n28 = Number To Fractional String(number=w139) -> (F-format string=w133:string)  [unwired: 3 in]
          n29 = Number To Fractional String(number=w137) -> (F-format string=w132:string)  [unwired: 3 in]
          n30 = Number To Fractional String(number=w138) -> (F-format string=w131:string)  [unwired: 3 in]
          n31 = Number To Fractional String(number=w136) -> (F-format string=w130:string)  [unwired: 3 in]
          n32 = Number To Fractional String(number=w135) -> (F-format string=w129:string)  [unwired: 3 in]
          n33 = Number To Fractional String(number=w134) -> (F-format string=w128:string)  [unwired: 3 in]
        }
      }
      n34 = case shown="3" w68 {
        tunnel: w69 -> [_ w84 w92 w108]
        tunnel: [w78 w81 w88 w103] -> w67
        tunnel: [w78 w80 w87 w102] -> w66
        tunnel: [w78 w79 w86 w101] -> w65
        tunnel: [w78 w79 w85 w100] -> w64
        tunnel: w63 -> [_ _ _ w99]
        tunnel: [w78 w79 w85 w95] -> w62
        tunnel: [w78 w79 w85 w94] -> w61
        tunnel: [w78 w79 w85 w93] -> w60
        frame 0, Default {
          w78 = "--"
        }
        frame 1 {
          w79 = "--"
          n35 = Unbundle By Name(w84) -> ("FREDDO resistomat.Res Ch1"=w82:dbl)
          n36 = Unbundle By Name(w84) -> ("FREDDO resistomat.tAMB"=w83:dbl)
          n37 = Number To Fractional String(number=w83) -> (F-format string=w81:string)  [unwired: 3 in]
          n38 = Number To Fractional String(number=w82) -> (F-format string=w80:string)  [unwired: 3 in]
        }
        frame 2 {
          w85 = "--"
          n39 = Unbundle By Name(w92) -> ("FREDDO resistomat.Res Ch1"=w90:dbl, "FREDDO resistomat.Res Ch2"=w89:dbl)
          n40 = Unbundle By Name(w92) -> ("FREDDO resistomat.tAMB"=w91:dbl)
          n41 = Number To Fractional String(number=w91) -> (F-format string=w88:string)  [unwired: 3 in]
          n42 = Number To Fractional String(number=w90) -> (F-format string=w87:string)  [unwired: 3 in]
          n43 = Number To Fractional String(number=w89) -> (F-format string=w86:string)  [unwired: 3 in]
        }
        frame 3 {
          n44 = Unbundle By Name(w108) -> ("FREDDO resistomat.tAMB"=w107:dbl)
          n45 = Unbundle By Name(w108) -> ("FREDDO resistomat.Res Ch1"=w106:dbl, "FREDDO resistomat.Res Ch2"=w105:dbl, "FREDDO resistomat.Res Ch3"=w104:dbl)
          n46 = Unbundle By Name(w99) -> ("Dt media"=w98:dbl, "Res media"=w97:dbl, "Res freddo media"=w96:dbl)
          n47 = Number To Fractional String(number=w107) -> (F-format string=w103:string)  [unwired: 3 in]
          n48 = Number To Fractional String(number=w106) -> (F-format string=w102:string)  [unwired: 3 in]
          n49 = Number To Fractional String(number=w105) -> (F-format string=w101:string)  [unwired: 3 in]
          n50 = Number To Fractional String(number=w104) -> (F-format string=w100:string)  [unwired: 3 in]
          n51 = Number To Fractional String(number=w98) -> (F-format string=w95:string)  [unwired: 3 in]
          n52 = Number To Fractional String(number=w97) -> (F-format string=w94:string)  [unwired: 3 in]
          n53 = Number To Fractional String(number=w96) -> (F-format string=w93:string)  [unwired: 3 in]
        }
      }
    }
    frame "RES METER - CONTINUO" {
      w142 = "--"
      w149 = "--"
      n54 = case shown="2" w147 {
        tunnel: w148 -> [_ w162 w170]
        tunnel: [w156 w159 w167] -> w145
        tunnel: [w156 w158 w166] -> w144
        tunnel: [w156 w157 "--"] -> w146
        tunnel: [w156 w157 w164] -> w143
        frame 0, Default {
          w156 = "--"
        }
        frame 1 {
          w157 = "--"
          n55 = Unbundle By Name(w162) -> ("FREDDO res meter.tAMB"=w161:dbl, "FREDDO res meter.Res Ch1"=w160:dbl)  [unwired: 1 out]
          n56 = Number To Fractional String(number=w161) -> (F-format string=w159:string)  [unwired: 3 in]
          n57 = Number To Fractional String(number=w160) -> (F-format string=w158:string)  [unwired: 3 in]
        }
        frame 2 {
          n58 = Unbundle By Name(w170) -> ("FREDDO res meter.tAMB"=w169:dbl, "FREDDO res meter.Res Ch1"=w168:dbl, "FREDDO res meter.Res Ch2"=w165:dbl)
          n59 = Number To Fractional String(number=w169) -> (F-format string=w167:string)  [unwired: 3 in]
          n60 = Number To Fractional String(number=w168) -> (F-format string=w166:string)  [unwired: 3 in]
          n61 = Number To Fractional String(number=w165) -> (F-format string=w164:string)  [unwired: 3 in]
        }
      }
      n62 = case shown="2" w155 {
        tunnel: w148 -> [_ w178 w188]
        tunnel: w154 -> [_ w177 w187]
        tunnel: [w171 w174 w184] -> w153
        tunnel: [w171 w173 w183] -> w152
        tunnel: [w171 w172 w181] -> w151
        tunnel: [w171 w172 w179] -> w150
        frame 0, Default {
          w171 = "--"
        }
        frame 1 {
          w172 = "--"
          n63 = Unbundle By Name(w178) -> ("Resistenze Res Meter.Res Ch1"=w176:dbl)
          n64 = Index Array(array=w177) -> (element=w175:dbl)  [unwired: 1 in]
          n65 = Number To Fractional String(number=w176) -> (F-format string=w174:string)  [unwired: 3 in]
          n66 = Number To Fractional String(number=w175) -> (F-format string=w173:string)  [unwired: 3 in]
        }
        frame 2 {
          n67 = Unbundle By Name(w188) -> ("Resistenze Res Meter.Res Ch1"=w186:dbl, "Resistenze Res Meter.Res Ch2"=w182:dbl)
          n68 = Index Array(array=w187) -> (element #1=w185:dbl, element #2=w180:dbl)  [unwired: 2 in]
          n69 = Number To Fractional String(number=w186) -> (F-format string=w184:string)  [unwired: 3 in]
          n70 = Number To Fractional String(number=w182) -> (F-format string=w181:string)  [unwired: 3 in]
          n71 = Number To Fractional String(number=w185) -> (F-format string=w183:string)  [unwired: 3 in]
          n72 = Number To Fractional String(number=w180) -> (F-format string=w179:string)  [unwired: 3 in]
        }
      }
    }
  }
  n73 = for {
    tunnel: w43 -> [w192] mode=indexing
    shift-right: [w193] -> w42
    shift-left: 0.0 -> [w190]
    tunnel: dbl[] [0.5, 1.0, 2.0, 4.0, 8.0, 16.0, 32.0, 64.0] -> [w191] mode=indexing
    n74 = Add(x=w190, y=w191) -> (x+y=w189:dbl)
    n75 = Select(t=w189, s=w192, f=w190) -> (s? t:f=w193:dbl)
  }
  n76 = Number To Fractional String(number="tamb") -> (F-format string=w49:string)  [unwired: 3 in]
  n77 = Unbundle By Name("MISURE ALL") -> ("MISURE WT"=w55:T5, "INTERFACCIA.AI.TENSIONI"=w33:T8[], "INTERFACCIA.AI.CORRENTI"=w32:T8[])
  n78 = global read "Global DATI MANUALI.vi" "DATI MANUALI TRASFORMATORE"() -> (w30:T36)
  n79 = global read "Global DATI MANUALI.vi" "INSERIMENTO DATI MANUALI?"() -> (w39:bool)
  n80 = global read "Global DATI MANUALI.vi" "DATI MANUALI GENERATORE"() -> (w36:T37)
  n81 = global read "Global DATI MANUALI.vi" "DATI MANUALI MOTORE DC"() -> (w37:cluster{"Vdinamo [V]":dbl})
  n82 = global read "Global DATI MANUALI.vi" "DATI MANUALI MOTORE AC"() -> (w35:T38)
  n83 = global read "Global DATI MANUALI.vi" "DATI MANUALI GENERICO"() -> (w38:T39)
  n84 = global read "Global DATI MANUALI.vi" "DATI MANUALI POMPA"() -> (w34:T40)
  n85 = case shown="\"AC MONOFASE\"" w5 {
    tunnel: "MISURE NM in" -> [w269 w337 w382 w425 w431 w432 w443 w479 w541 w625]
    tunnel: w55 -> [w221 w336 w340 w426 _ _ _ w480 w572 w591]
    tunnel: [w250 w315 w381 w410 w431 w432 w442 w478 w540 w606] -> w57
    tunnel: [w229 w295 _ w400 _ _ _ w452 _ w600] -> w56
    tunnel: "MISURE ALL" -> [_ _ _ w406 _ _ _ _ _ _]
    tunnel: w49 -> [w198 w314 _ _ _ _ _ _ _ w584]
    tunnel: "RPM" -> [w245 w311 _ _ _ _ _ _ _ _]
    tunnel: "Cluster INFO" -> [w247 w300 _ _ _ _ _ _ _ _]
    tunnel: [w232 w296 _ _ _ _ _ _ _ _] -> w47
    tunnel: w42 -> [_ w292 _ _ _ _ _ _ _ _]
    tunnel: w39 -> [w220 _ w339 _ _ _ w433 w477 w526 w590]
    tunnel: w38 -> [_ _ _ _ _ _ w444 _ _ _]
    tunnel: w37 -> [_ _ _ w409 _ _ _ _ _ _]
    tunnel: w36 -> [_ _ _ _ _ _ _ w476 w539 _]
    tunnel: w35 -> [w219 _ _ _ _ _ _ _ _ _]
    tunnel: w34 -> [_ _ _ _ _ _ _ _ _ w585]
    tunnel: w33 -> [_ _ w380 _ _ _ _ _ _ _]
    tunnel: w32 -> [_ _ w347 _ _ _ _ _ _ _]
    tunnel: w30 -> [_ _ w338 _ _ _ _ _ _ _]
    tunnel: w23 -> [w208 w290 _ _ _ _ _ _ _ w583]
    tunnel: w22 -> [w207 w289 _ _ _ _ _ _ _ _]
    tunnel: w21 -> [w206 _ _ _ _ _ _ _ _ _]
    tunnel: w20 -> [w205 w288 _ _ _ _ _ _ _ w582]
    tunnel: w19 -> [w204 w287 _ _ _ _ _ _ _ _]
    tunnel: w18 -> [w203 _ _ _ _ _ _ _ _ _]
    tunnel: w14 -> [w202 w286 _ _ _ _ _ _ _ w581]
    tunnel: w13 -> [w201 w285 _ _ _ _ _ _ _ w580]
    tunnel: w12 -> [w200 w284 _ _ _ _ _ _ _ _]
    tunnel: w11 -> [w199 _ _ _ _ _ _ _ _ _]
    tunnel: w3 -> [w197 _ _ _ _ _ _ _ _ _]
    tunnel: w2 -> [w196 _ _ _ _ _ _ _ _ _]
    tunnel: w1 -> [w195 _ _ _ _ _ _ _ _ _]
    frame "AC TRIFASE", Default {
      # "trifase 3 canali + FRENO"
      n86 = case shown="True" w220 {
        tunnel: [w276 w282] -> w227
        tunnel: [w275 w277] -> w226
        tunnel: [w274 w278] -> w225
        tunnel: [w273 w279] -> w224
        tunnel: [w272 w280] -> w223
        tunnel: [w271 w281] -> w222
        tunnel: w221 -> [w270 _]
        tunnel: w219 -> [_ w283]
        frame False {
          n87 = Unbundle By Name(w270) -> ("URMS 1"=w276:dbl, "URMS 2"=w275:dbl, "URMS 3"=w274:dbl, "IRMS 1"=w273:dbl, "IRMS 2"=w272:dbl, "IRMS 3"=w271:dbl)
        }
        frame True {
          n88 = Unbundle By Name(w283) -> ("U1 [V]"=w282:dbl, "U2 [V]"=w277:dbl, "U3 [V]"=w278:dbl, "I1 [A]"=w279:dbl, "I2 [A]"=w280:dbl, "I3 [A]"=w281:dbl)
        }
      }
      n89 = Unbundle By Name(w247) -> ("Dati targa motore.Npoli"=w246:dbl, "Dati targa motore.Vnom"=w240:dbl, "Dati targa motore.Inom"=w239:dbl)
      n90 = Absolute Value(x=w245) -> (abs(x)=w194:dbl)
      n91 = Unbundle By Name(w221) -> ("F U 1"=w244:dbl, "URMS SIGMA"=w232:dbl, "IRMS SIGMA"=w241:dbl, "P SIGMA"=w229:dbl, "S SIGMA"=w217:dbl, "Q SIGMA"=w214:dbl)
      n92 = call "Calcolo SCORRIMENTO.vi"("POLI"=w246, "FREQ"=w244, "RPM"=w194) -> ("SCORRIMENTO"=w249:dbl)  [unwired: 8 in]
      n93 = Divide(x=w229, y=w217) -> (x/y=w228:dbl)
      n94 = Divide(x=w229, y=1000.0) -> (x/y=w260:dbl)
      n95 = Divide(x=w217, y=1000.0) -> (x/y=w216:dbl)
      n96 = Divide(x=w214, y=1000.0) -> (x/y=w213:dbl)
      n97 = call "ricalcolo grandezze.vi"("^2?"=FALSE, "grandezza nom"=w239, "V"=w232, "Vn"=w240, "grandezza"=w241) -> ("grandezza ric. /nom."=w235:dbl, "grandezza ric."=w237:dbl)  [unwired: 5 in]
      n98 = call "Calcolo sbilanciamento.vi"("Numeric 1"=w222, "Numeric 2"=w223, "Numeric 3"=w224) -> ("sbil%"=w231:dbl)  [unwired: 8 in]
      n99 = Build Array(w244, w232, w241, w229, w260, w228, w227, w226, w225, w224, w223, w222, w231, w217, w216, w214, w213) -> (w268:dbl[])
      n100 = Number To Fractional String(number=w268, precision (6)=i16 5) -> (F-format string=w267:string[])  [unwired: 2 in]
      n101 = Number To Fractional String(number=w237, precision (6)=i16 5) -> (F-format string=w234:string)  [unwired: 2 in]
      n102 = Number To Fractional String(number=w235, precision (6)=i16 5) -> (F-format string=w233:string)  [unwired: 2 in]
      n103 = Number To Fractional String(number=w249, precision (6)=i16 5) -> (F-format string=w243:string)  [unwired: 2 in]
      n104 = Index Array(array=w267) -> (element #1=w266:string, element #2=w265:string, element #3=w264:string, element #4=w263:string, element #5=w252:string, element #6=w253:string, element #7=w254:string, element #8=w255:string, element #9=w256:string, element #10=w257:string, element #11=w258:string, element #12=w259:string, element #13=w230:string, element #14=w212:string, element #15=w211:string, element #16=w210:string, element #17=w209:string)  [unwired: 17 in]
      n105 = Bundle By Name(cluster=w269, "f [Hz]"=w266, "U123_media [V]"=w265, "I123_media [A]*I"=w264, "P1 [W]"=w263, "P1 [kW]"=w252, "pf"=w253, "U1[V]"=w254, "U2 [V]"=w255, "U3 [V]"=w256, "I1[A]"=w257, "I2[A]"=w258, "I3[A]"=w259, "I_123_sbil [%]"=w230, "Scorr[%]"=w243, "Iric[A]"=w234, "Iric\\Inom"=w233, "S [VA]"=w212, "S [kVA]"=w211, "Q [VAR]"=w210, "Q [kVAR]"=w209) -> (w251:T31)
      n106 = Bundle By Name(cluster=w251, "R1[ohm]"=w208, "R2[ohm]"=w207, "R3[ohm]"=w206, "DT_R1[°C]"=w205, "DT_R2[°C]"=w204, "DT_R3[°C]"=w203, "Tamb[°C]"=w198, "TambFreddo[°C]"=w202, "R1_freddo[ohm]"=w201, "R2_freddo[ohm]"=w200, "R3_freddo[ohm]"=w199, "Rmedia_freddo[ohm]"=w197, "Rmedia[ohm]"=w196, "DT_media[°C]"=w195) -> (w250:T31)
    }
    frame "AC MONOFASE" {
      # "canale 1 linea?"
      # "MONOFASE"
      n107 = Unbundle By Name(w300) -> ("Dati targa motore.Npoli"=w309:dbl)
      n108 = Unbundle By Name(w300) -> ("Dati targa motore.Vnom"=w305:dbl, "Dati targa motore.Inom"=w307:dbl)
      n109 = Unbundle By Name(w336) -> ("F U 1"=w310:dbl, "URMS 3"=w296:dbl, "URMS 2"=w335:dbl, "URMS 1"=w325:dbl, "IRMS 1"=w299:dbl, "IRMS 3"=w324:dbl, "IRMS 2"=w323:dbl, "P 3"=w295:dbl, "S 3"=w294:dbl)
      n110 = call "Calcolo SCORRIMENTO.vi"("POLI"=w309, "FREQ"=w310, "RPM"=w311) -> ("SCORRIMENTO"=w313:dbl)  [unwired: 8 in]
      n111 = Divide(x=w295, y=w294) -> (x/y=w293:dbl)
      n112 = Divide(x=w295, y=1000.0) -> (x/y=w317:dbl)
      n113 = call "ricalcolo grandezze.vi"("^2?"=FALSE, "grandezza nom"=w307, "V"=w296, "Vn"=w305, "grandezza"=w299) -> ("grandezza ric. /nom."=w301:dbl, "grandezza ric."=w303:dbl)  [unwired: 5 in]
      n114 = Build Array(w310, w296, w335, w325, w299, w324, w323, w295, w317, w293) -> (w334:dbl[])
      n115 = Number To Fractional String(number=w334, precision (6)=i16 5) -> (F-format string=w333:string[])  [unwired: 2 in]
      n116 = Number To Fractional String(number=w292) -> (F-format string=w291:string)  [unwired: 3 in]
      n117 = Index Array(array=w333) -> (element #1=w332:string, element #2=w331:string, element #3=w330:string, element #4=w329:string, element #5=w328:string, element #6=w327:string, element #7=w326:string, element #8=w322:string, element #9=w321:string, element #10=w320:string)  [unwired: 10 in]
      n118 = Number To Fractional String(number=w313, precision (6)=i16 5) -> (F-format string=w308:string)  [unwired: 2 in]
      n119 = Number To Fractional String(number=w303, precision (6)=i16 5) -> (F-format string=w298:string)  [unwired: 2 in]
      n120 = Number To Fractional String(number=w301, precision (6)=i16 5) -> (F-format string=w297:string)  [unwired: 2 in]
      n121 = Bundle By Name(cluster=w337, "f [Hz]"=w332, "Ulin[V]"=w331, "Uaux [V]"=w330, "Uc [V]"=w329, "Ilin[A]*I"=w328, "Imar[A]"=w327, "Iaux[A]"=w326, "P1 [W]"=w322, "P1 [kW]"=w321, "pf"=w320, "Scorr[%]"=w308, "Iric[A]"=w298, "Iric\\Inom"=w297, "Cond[uF]"=w291) -> (w316:T31)
      n122 = Bundle By Name(cluster=w316, "R_marcia[ohm]"=w290, "R_aux[ohm]"=w289, "DT_marcia[°C]"=w288, "DT_aux[°C]"=w287, "Tamb[°C]"=w314, "TambFreddo[°C]"=w286, "R_Marcia_freddo[ohm]"=w285, "R_Aux_freddo[ohm]"=w284) -> (w315:T31)
    }
    frame "TRASFORMATORE" {
      w348 = 0.0 ("element")
      # "TRASFORMATORE"
      n123 = case shown="True" w339 {
        tunnel: [w392 w395] -> w343
        tunnel: [w391 w394] -> w342
        tunnel: [w390 w393] -> w341
        tunnel: w340 -> [w389 _]
        tunnel: w338 -> [_ w396]
        frame False {
          n124 = Unbundle By Name(w389) -> ("IRMS 1"=w392:dbl, "IRMS 2"=w391:dbl, "IRMS 3"=w390:dbl)
        }
        frame True {
          n125 = Unbundle By Name(w396) -> ("I1 [A]"=w395:dbl, "I2 [A]"=w394:dbl, "I3 [A]"=w393:dbl)
        }
      }
      n126 = Unbundle By Name(w340) -> ("F U 1"=w369:dbl, "P SIGMA"=w368:dbl, "LAMBDA SIGMA"=w367:dbl)  [unwired: 3 out]
      n127 = Unbundle By Name(w340) -> ("URMS 1"=w385:dbl, "URMS 2"=w384:dbl, "URMS 3"=w383:dbl)
      n128 = Index Array(array=w380) -> (element #1=w379:T8, element #2=w378:T8, element #3=w377:T8)  [unwired: 3 in]
      n129 = Index Array(array=w347) -> (element #1=w346:T8, element #2=w345:T8, element #3=w344:T8)  [unwired: 3 in]
      n130 = Unbundle By Name(w379) -> ("Misura"=w376:dbl)
      n131 = Unbundle By Name(w378) -> ("Misura"=w375:dbl)
      n132 = Unbundle By Name(w377) -> ("Misura"=w374:dbl)
      n133 = Unbundle By Name(w346) -> ("Misura"=w373:dbl)
      n134 = Unbundle By Name(w345) -> ("Misura"=w372:dbl)
      n135 = Unbundle By Name(w344) -> ("Misura"=w371:dbl)
      n136 = Build Array(w376, w375, w374, w373, w372, w371) -> (w370:dbl[])
      n137 = Build Array (concatenate)(w370, w385, w384, w383, w348, w348, w348, w343, w342, w341, w369, w368, w367) -> (w388:dbl[])
      n138 = Number To Fractional String(number=w388, precision (6)=i16 5) -> (F-format string=w387:string[])  [unwired: 2 in]
      n139 = Index Array(array=w387) -> (element #1=w366:string, element #2=w365:string, element #3=w364:string, element #4=w363:string, element #5=w362:string, element #6=w361:string, element #7=w360:string, element #8=w359:string, element #9=w358:string, element #10=w357:string, element #11=w356:string, element #12=w355:string, element #13=w354:string, element #14=w353:string, element #15=w352:string, element #16=w351:string, element #17=w350:string, element #18=w349:string)  [unwired: 21 in, 3 out]
      n140 = Bundle By Name(cluster=w382, "U1'[V]"=w366, "U2'[V]"=w365, "U3'[V]"=w364, "I1'[A]"=w363, "I2'[A]"=w362, "I3'[A]"=w361, "U''R-N"=w360, "U''S-N"=w359, "U'' T-N"=w358, "U''R-S"=w357, "U''R-T"=w356, "U''S-T"=w355, "I1''[A]"=w354, "I2''[A]"=w353, "I3''[A]"=w352, "F''[Hz]"=w351, "P''[kW]"=w350, "CosFi''"=w349) -> (w381:T31)
    }
    frame "DC ECCITAZIONE" {
      # "DC CON ECCITAZIONE+FRENO \\ MOTORE CC"
      n141 = Unbundle By Name(w406) -> ("DCREG.Parametri di misura.M018"=w405:dbl)
      n142 = Unbundle By Name(w409) -> ("Vdinamo [V]"=w408:dbl)
      n143 = Unbundle By Name(w426) -> ("URMS 3"=w399:dbl, "URMS 2"=w403:dbl, "IRMS 3"=w398:dbl)  [unwired: 3 out]
      n144 = Divide(x=w405, y=100.0) -> (x/y=w402:dbl)
      n145 = Multiply(x=w399, y=w398) -> (x*y=w397:dbl)
      n146 = Multiply(x=w403, y=w402) -> (x*y=w401:dbl)
      n147 = Divide(x=w401, y=1000.0) -> (x/y=w417:dbl)
      n148 = Divide(x=w401, y=1000.0) -> (x/y=w416:dbl)
      n149 = Add(x=w417, y=w416) -> (x+y=w415:dbl)
      n150 = Add(x=w397, y=w401) -> (x+y=w400:dbl)
      n151 = Build Array(w399, w403, w398, w402, w397, w401, w417, w416, w400, w415, w408) -> (w430:dbl[])
      n152 = Number To Fractional String(number=w430, precision (6)=i16 5) -> (F-format string=w429:string[])  [unwired: 2 in]
      n153 = Index Array(array=w429) -> (element #1=w424:string, element #2=w423:string, element #3=w422:string, element #4=w421:string, element #5=w420:string, element #6=w419:string, element #7=w414:string, element #8=w413:string, element #9=w412:string, element #10=w411:string, element #11=w407:string)  [unwired: 11 in]
      n154 = Bundle By Name(cluster=w425, "Uarm[V]"=w424, "Uecc[V]"=w423, "Iarm[A]*I"=w422, "Iecc[A]"=w421, "P1arm[W]"=w420, "P1ecc[W]"=w419, "Parm[kW]"=w414, "P1ecc[kW]"=w413, "P1 [W]"=w412, "P1 [kW]"=w411, "V dinamo[V]"=w407) -> (w410:T31)
    }
    frame "DC NO ECCITAZIONE" {
      # "DC NO ECCITAZIONE"
    }
    frame "POMPA MONOFASE" {
    }
    frame "GENERICO" {
      # "GENERICO"
      n155 = case shown="True" w433 {
        tunnel: w444 -> [_ w451]
        tunnel: [_ w450] -> w441
        frame False {
        }
        frame True {
          n156 = Unbundle By Name(w451) -> ("Tensione [V]"=w449:dbl, "Corrente [A]"=w448:dbl, "Frequenza [Hz]"=w447:dbl, "Velocità [RPM]"=w446:dbl, "I saldatura [A]"=w445:dbl)
          n157 = Build Array(w449, w448, w447, w446, w445) -> (w450:dbl[])
        }
      }
      n158 = Number To Fractional String(number=w441, precision (6)=i16 5) -> (F-format string=w440:string[])  [unwired: 2 in]
      n159 = Index Array(array=w440) -> (element #1=w438:string, element #2=w437:string, element #3=w436:string, element #4=w435:string, element #5=w434:string)  [unwired: 5 in]
      n160 = Bundle By Name(cluster=w443, "U123_media [V]"=w438, "I123_media [A]*I"=w437, "f [Hz]"=w436, "n [rpm]"=w435, "f [Hz]"=w434) -> (w442:T31)
    }
    frame "ALTERNATORE TRASCINATO" {
      # "FRENO TRASCIN + AFE \\ ALTERNATORE"
      n161 = Unbundle By Name(w480) -> ("F U 1"=w489:dbl, "URMS SIGMA"=w488:dbl, "IRMS SIGMA"=w487:dbl, "P SIGMA"=w452:dbl, "S SIGMA"=w459:dbl, "Q SIGMA"=w462:dbl, "LAMBDA SIGMA"=w453:dbl)
      n162 = Divide(x=w452, y=w459) -> ()  [unwired: 1 out]
      n163 = case shown="True" w477 {
        tunnel: w476 -> [_ w515]
        tunnel: [_ w514] -> w475
        tunnel: [_ w513] -> w474
        tunnel: [_ w512] -> w473
        tunnel: [_ w511] -> w472
        tunnel: [_ w510] -> w471
        tunnel: [_ w509] -> w470
        frame False {
        }
        frame True {
          n164 = Unbundle By Name(w515) -> ("ECCITATRICE.VDC [V]"=w514:dbl, "ECCITATRICE.IDC [A]"=w513:dbl, "ROTORE.Vdc [V]"=w512:dbl, "ROTORE.Idc [A]"=w511:dbl, "ROTORE.Vac [V]"=w510:dbl, "ROTORE.Iac [A]"=w509:dbl)
        }
      }
      n165 = Divide(x=w452, y=1000.0) -> (x/y=w500:dbl)
      n166 = Divide(x=w459, y=1000.0) -> (x/y=w458:dbl)
      n167 = Divide(x=w462, y=1000.0) -> (x/y=w463:dbl)
      n168 = Unbundle By Name(w480) -> ("URMS 1"=w486:dbl, "URMS 2"=w485:dbl, "URMS 3"=w484:dbl, "IRMS 1"=w483:dbl, "IRMS 2"=w482:dbl, "IRMS 3"=w481:dbl)
      n169 = call "Calcolo sbilanciamento.vi"("Numeric 1"=w481, "Numeric 2"=w482, "Numeric 3"=w483) -> ("sbil%"=w491:dbl)  [unwired: 8 in]
      n170 = Build Array(w489, w488, w487, w452, w500, w453, w486, w485, w484, w483, w482, w481, w491, w475, w474, w473, w472, w471, w470, w462, w463, w459, w458) -> (w508:dbl[])
      n171 = Number To Fractional String(number=w508, precision (6)=i16 5) -> (F-format string=w507:string[])  [unwired: 2 in]
      n172 = Index Array(array=w507) -> (element #1=w506:string, element #2=w505:string, element #3=w504:string, element #4=w503:string, element #5=w492:string, element #6=w493:string, element #7=w494:string, element #8=w495:string, element #9=w496:string, element #10=w497:string, element #11=w498:string, element #12=w499:string, element #13=w490:string, element #14=w469:string, element #15=w468:string, element #16=w467:string, element #17=w466:string, element #18=w465:string, element #19=w464:string, element #20=w457:string, element #21=w456:string, element #22=w455:string, element #23=w454:string)  [unwired: 24 in, 1 out]
      n173 = Bundle By Name(cluster=w479, "f [Hz]"=w506, "U123_media [V]"=w505, "I123_media [A]*I"=w504, "P1 [W]"=w503, "P1 [kW]"=w492, "pf"=w493, "U1[V]"=w494, "U2 [V]"=w495, "U3 [V]"=w496, "I1[A]"=w497, "I2[A]"=w498, "I3[A]"=w499, "I_123_sbil [%]"=w490, "Vdc eccitatrice[V]"=w469, "Idc eccitatrice[A]"=w468, "Vdc rotore[V]"=w467, "Idc rotore[A]"=w466, "Vac rotore[V]"=w465, "Iac rotore[V]"=w464, "Q [VAR]"=w457, "Q [kVAR]"=w456, "S [VA]"=w455, "S [kVA]"=w454) -> (w478:T31)
    }
    frame "GRUPPO ELETTROGENO" {
      # "CARICO RESISTIVO - GRUPPO ELETTROGENO"
      n174 = case shown="True" w526 {
        tunnel: w539 -> [_ w579]
        tunnel: [_ w578] -> w538
        tunnel: [_ w577] -> w537
        tunnel: [_ w576] -> w536
        tunnel: [_ w575] -> w535
        tunnel: [_ w574] -> w534
        tunnel: [_ w573] -> w533
        frame False {
        }
        frame True {
          n175 = Unbundle By Name(w579) -> ("ECCITATRICE.VDC [V]"=w578:dbl, "ECCITATRICE.IDC [A]"=w577:dbl, "ROTORE.Vdc [V]"=w576:dbl, "ROTORE.Idc [A]"=w575:dbl, "ROTORE.Vac [V]"=w574:dbl, "ROTORE.Iac [A]"=w573:dbl)
        }
      }
      n176 = Unbundle By Name(w572) -> ("F U 1"=w551:dbl, "URMS SIGMA"=w550:dbl, "IRMS SIGMA"=w549:dbl, "P SIGMA"=w548:dbl, "S SIGMA"=w521:dbl, "Q SIGMA"=w524:dbl)
      n177 = Divide(x=w548, y=w521) -> (x/y=w552:dbl)
      n178 = Divide(x=w548, y=1000.0) -> (x/y=w563:dbl)
      n179 = Divide(x=w521, y=1000.0) -> (x/y=w520:dbl)
      n180 = Divide(x=w524, y=1000.0) -> (x/y=w523:dbl)
      n181 = Unbundle By Name(w572) -> ("URMS 1"=w547:dbl, "URMS 2"=w546:dbl, "URMS 3"=w545:dbl, "IRMS 1"=w544:dbl, "IRMS 2"=w543:dbl, "IRMS 3"=w542:dbl)
      n182 = call "Calcolo sbilanciamento.vi"("Numeric 1"=w542, "Numeric 2"=w543, "Numeric 3"=w544) -> ("sbil%"=w554:dbl)  [unwired: 8 in]
      n183 = Build Array(w551, w550, w549, w548, w563, w552, w547, w546, w545, w544, w543, w542, w554, w538, w537, w536, w535, w534, w533, w524, w523, w521, w520) -> (w571:dbl[])
      n184 = Number To Fractional String(number=w571, precision (6)=i16 5) -> (F-format string=w570:string[])  [unwired: 2 in]
      n185 = Index Array(array=w570) -> (element #1=w569:string, element #2=w568:string, element #3=w567:string, element #4=w566:string, element #5=w555:string, element #6=w556:string, element #7=w557:string, element #8=w558:string, element #9=w559:string, element #10=w560:string, element #11=w561:string, element #12=w562:string, element #13=w553:string, element #14=w532:string, element #15=w531:string, element #16=w530:string, element #17=w529:string, element #18=w528:string, element #19=w527:string, element #20=w519:string, element #21=w518:string, element #22=w517:string, element #23=w516:string)  [unwired: 23 in]
      n186 = Bundle By Name(cluster=w541, "f [Hz]"=w569, "U123_media [V]"=w568, "I123_media [A]*I"=w567, "P1 [W]"=w566, "P1 [kW]"=w555, "pf"=w556, "U1[V]"=w557, "U2 [V]"=w558, "U3 [V]"=w559, "I1[A]"=w560, "I2[A]"=w561, "I3[A]"=w562, "I_123_sbil [%]"=w553, "Vdc eccitatrice[V]"=w532, "Idc eccitatrice[A]"=w531, "Vdc rotore[V]"=w530, "Idc rotore[A]"=w529, "Vac rotore[V]"=w528, "Iac rotore[V]"=w527, "Q [VAR]"=w519, "Q [kVAR]"=w518, "S [VA]"=w517, "S [kVA]"=w516) -> (w540:T31)
    }
    frame "POMPA TRIFASE" {
      # "AC TRIFASE - POMPA"
      n187 = case shown="False" w590 {
        tunnel: [w632 w640] -> w597
        tunnel: [w631 w635] -> w596
        tunnel: [w630 w636] -> w595
        tunnel: [w629 w637] -> w594
        tunnel: [w628 w638] -> w593
        tunnel: [w627 w639] -> w592
        tunnel: w591 -> [w626 _]
        tunnel: w585 -> [_ w641]
        tunnel: [_ w634] -> w589
        tunnel: [_ w633] -> w588
        frame False {
          n188 = Unbundle By Name(w626) -> ("URMS 1"=w632:dbl, "URMS 2"=w631:dbl, "URMS 3"=w630:dbl, "IRMS 1"=w629:dbl, "IRMS 2"=w628:dbl, "IRMS 3"=w627:dbl)
        }
        frame True {
          n189 = Unbundle By Name(w641) -> ("U1 [V]"=w640:dbl, "U2 [V]"=w635:dbl, "U3 [V]"=w636:dbl, "I1 [A]"=w637:dbl, "I2 [A]"=w638:dbl, "I3 [A]"=w639:dbl, "Q"=w634:dbl, "H"=w633:dbl)
        }
      }
      n190 = Unbundle By Name(w591) -> ("F U 1"=w605:dbl, "URMS SIGMA"=w603:dbl, "IRMS SIGMA"=w604:dbl, "P SIGMA"=w600:dbl, "S SIGMA"=w599:dbl)
      n191 = Divide(x=w600, y=w599) -> (x/y=w598:dbl)
      n192 = Divide(x=w600, y=1000.0) -> (x/y=w616:dbl)
      n193 = call "Calcolo sbilanciamento.vi"("Numeric 1"=w592, "Numeric 2"=w593, "Numeric 3"=w594) -> ("sbil%"=w602:dbl)  [unwired: 8 in]
      n194 = Build Array(w605, w603, w604, w600, w616, w598, w597, w596, w595, w594, w593, w592, w602, w589, w588) -> (w624:dbl[])
      n195 = Number To Fractional String(number=w624, precision (6)=i16 5) -> (F-format string=w623:string[])  [unwired: 2 in]
      n196 = Index Array(array=w623) -> (element #1=w622:string, element #2=w621:string, element #3=w620:string, element #4=w619:string, element #5=w608:string, element #6=w609:string, element #7=w610:string, element #8=w611:string, element #9=w612:string, element #10=w613:string, element #11=w614:string, element #12=w615:string, element #13=w601:string, element #14=w587:string, element #15=w586:string)  [unwired: 15 in]
      n197 = Bundle By Name(cluster=w625, "f [Hz]"=w622, "U123_media [V]"=w621, "I123_media [A]*I"=w620, "P1 [W]"=w619, "P1 [kW]"=w608, "pf"=w609, "U1[V]"=w610, "U2 [V]"=w611, "U3 [V]"=w612, "I1[A]"=w613, "I2[A]"=w614, "I3[A]"=w615, "I_123_sbil [%]"=w601, "Portata Q"=w587, "Pressione H"=w586) -> (w607:T31)
      n198 = Bundle By Name(cluster=w607, "R1[ohm]"=w583, "DT_R1[°C]"=w582, "Tamb[°C]"=w584, "TambFreddo[°C]"=w581, "R1_freddo[ohm]"=w580) -> (w606:T31)
    }
  }
  "MISURE NM out" <- w57
  "P1[W]" <- w56
  "V" <- w47
